vi "Safety_Check.vi"(0 "Duty No":u16 format="%.0b", 1 "Values":dbl[](array[numeric]) format="%.2f", 2 "Ch Names":string[](array[string]), 3 "Adam Loop Count":i32, 4 "Current Time":dbl) -> (5 "Scan comment":string)   [LabVIEW 2022 SP3]
uses:
  ADAM Client/Sub VIs/ADAM Controls/Update_scan_value.ctl
  Anemometry/Anemometry Sub Vis/Controls/In_Range.ctl
  ADAM Client/Sub VIs/Channel_State_Control.ctl
  Anemometry/Anemometry Sub Vis/Globals/Gas_management_global.vi
  ADAM_Global.vi
  Anemometry/Anemometry Sub Vis/Globals/EnFlo_Tunnel_Global.vi
panel:
  in  "Valve Tolerance":dbl=0.07
  in  "Minimum St Dev for Ozone inst":dbl=0.3
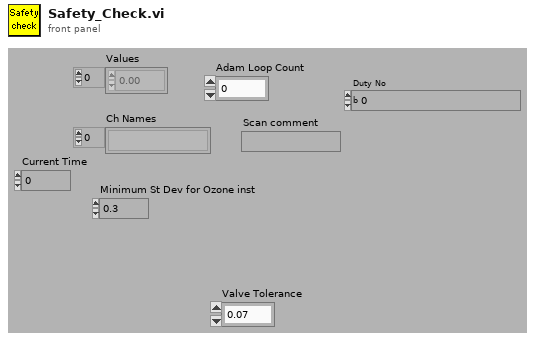
[diagram p1: front panel]
types:
  T1 = typedef "Update_scan_value.ctl" = cluster{"Channel Name":string, "New Value":dbl, "!Auto_Off":bool}
  T2 = enum16{"Append to Global", "Read Global then Clear"}
  T3 = enum16{"On", "Off", "Always On", "Always Off", "Delete"}
  T4 = typedef "In_Range.ctl" = enum16{"%", "±", "% & ±"}
  T5 = typedef "Channel_State_Control.ctl" = enum16{"Channel Name", "Channel Name Starts with", "Main Address"}
  T6 = cluster{"Bus Bar":string, "Connected Items":string[]}
  T7 = cluster{"Bus Bar":string, "Connected Items":string[]}[]
  T8 = typedef "LVDateTimeRec.ctl" = cluster{"fractional second":dbl, "second":i32, "minute":i32, "hour":i32, "day of month":i32, "month":i32, "year":i32, "day of week":i32, "day of year":i32, "DST":i32}
  T9 = typedef "Ch_description_ADAM.ctl" = cluster{"Ch Name":string, "Type":T10, "Function":T11, "Ch State":T12, "Calibration type":T13, "A":dbl, "B":dbl, "C":dbl, "D":dbl, "Comments":string, "Address":T14, "String":string, "Duty":u16}
  T10 = typedef "Module_type_ADAM.ctl" = string
  T11 = typedef "Function_ADAM.ctl" = enum16{"Analogue Input", "Digital Input", "Event counter", "Event rate", "Analogue Output", "Digital Output", "Relay Output"}
  T12 = typedef "Channel_State.ctl" = enum16{"On", "Off", "Always On", "Always Off"}
  T13 = typedef "Calib_type_ADAM.ctl" = string
  T14 = typedef "Address.ctl" = cluster{"Main":i32, "Ch.":i32, "Sub":i32, "Port Name":string}
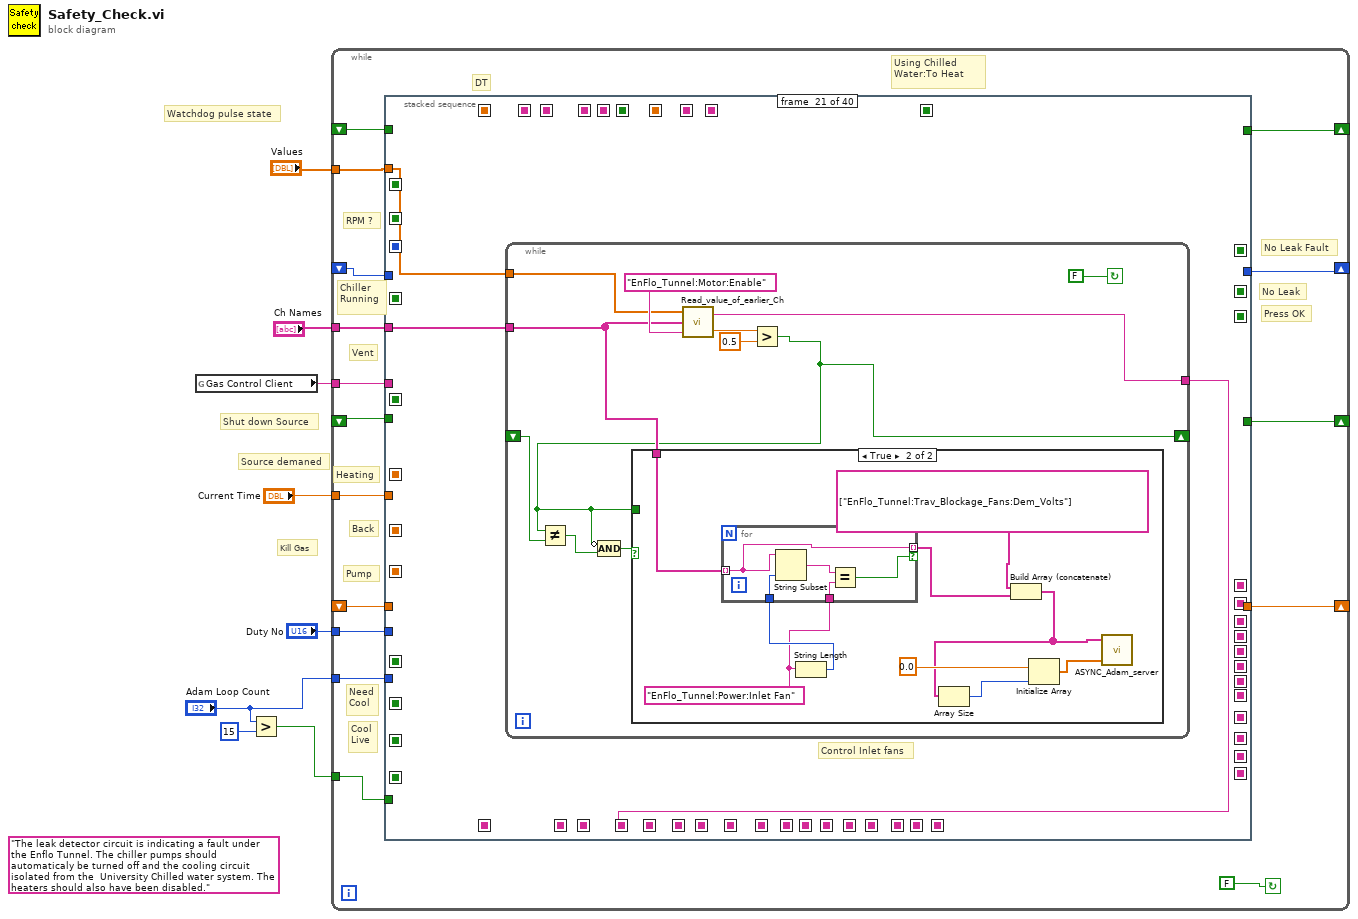
[diagram p0: block diagram]
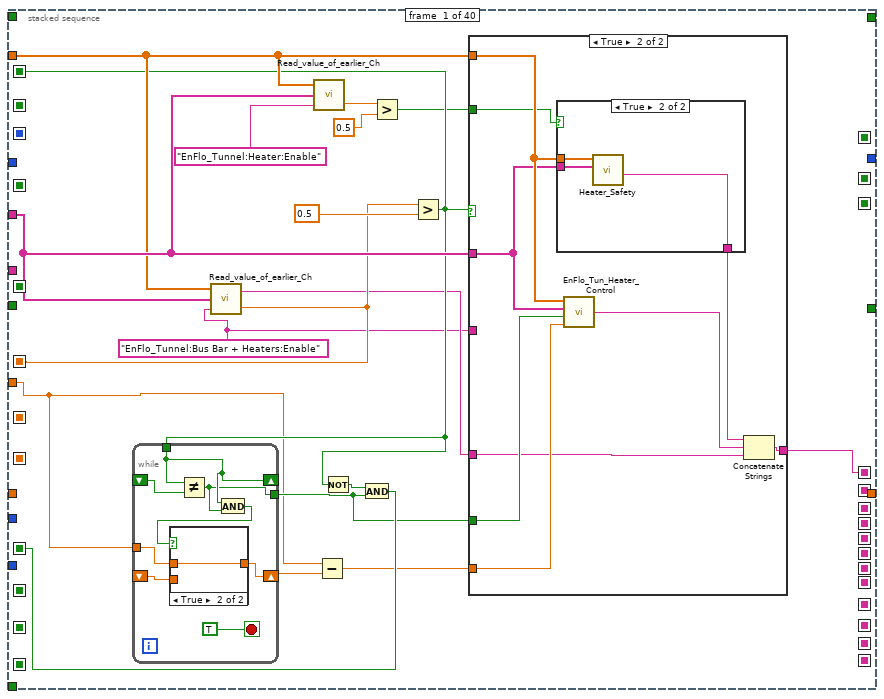
[diagram p2: hidden frame]
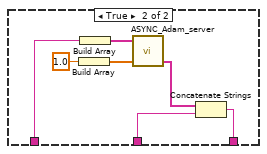
[diagram p5: hidden frame]
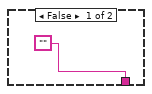
[diagram p6: hidden frame]
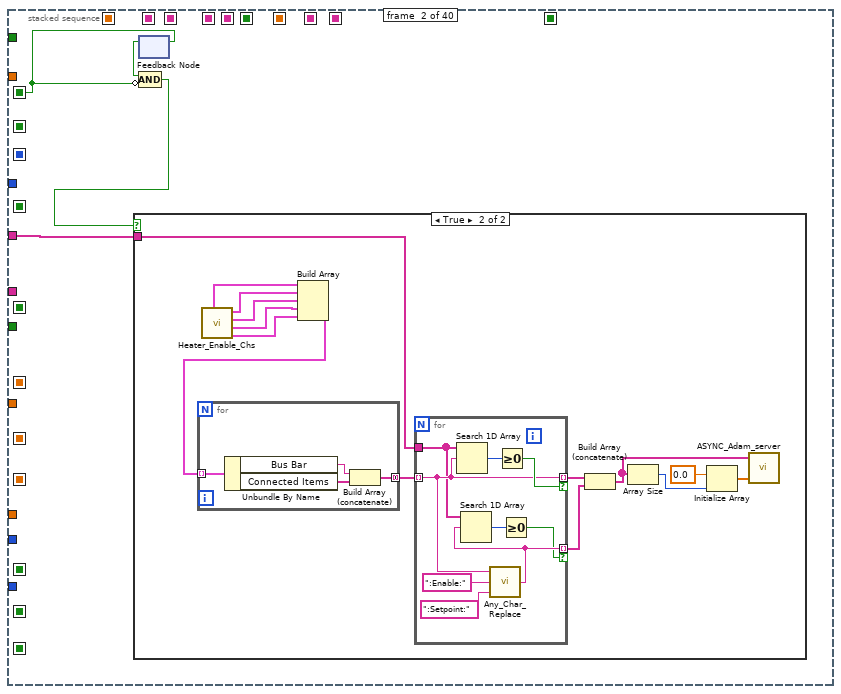
[diagram p7: hidden frame]
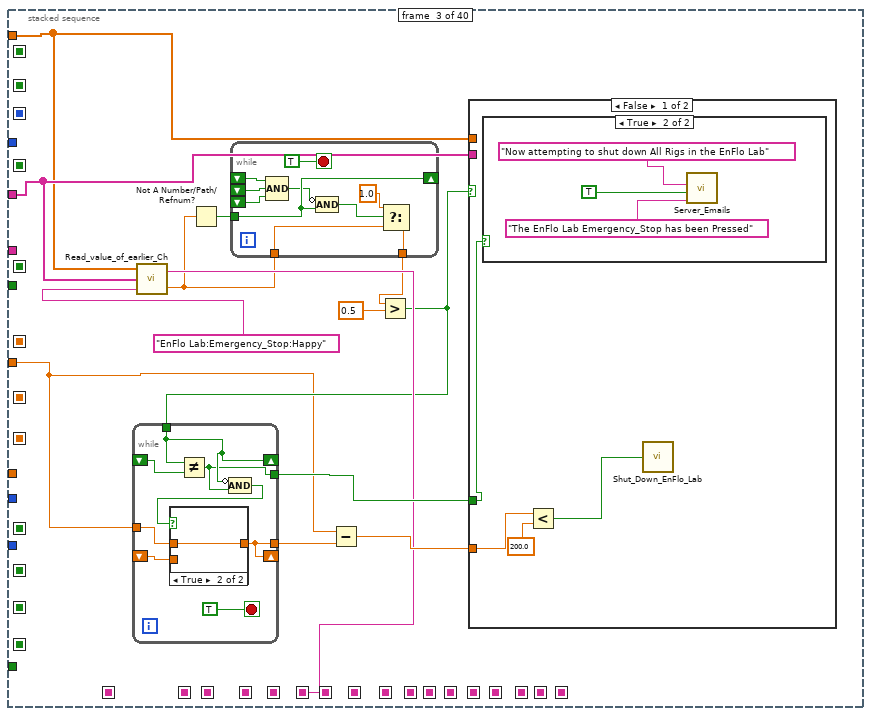
[diagram p9: hidden frame]
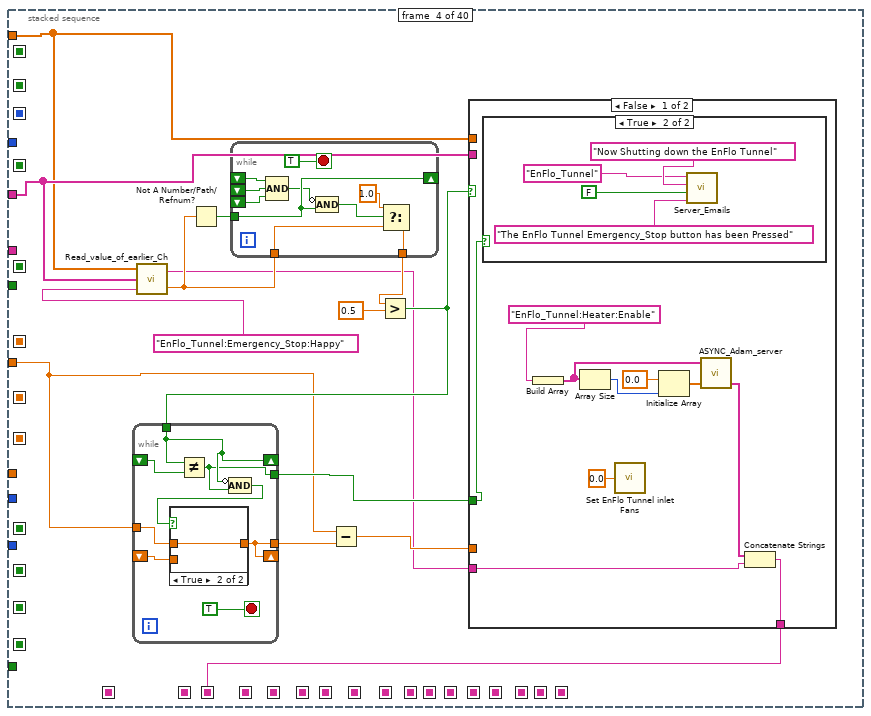
[diagram p13: hidden frame]
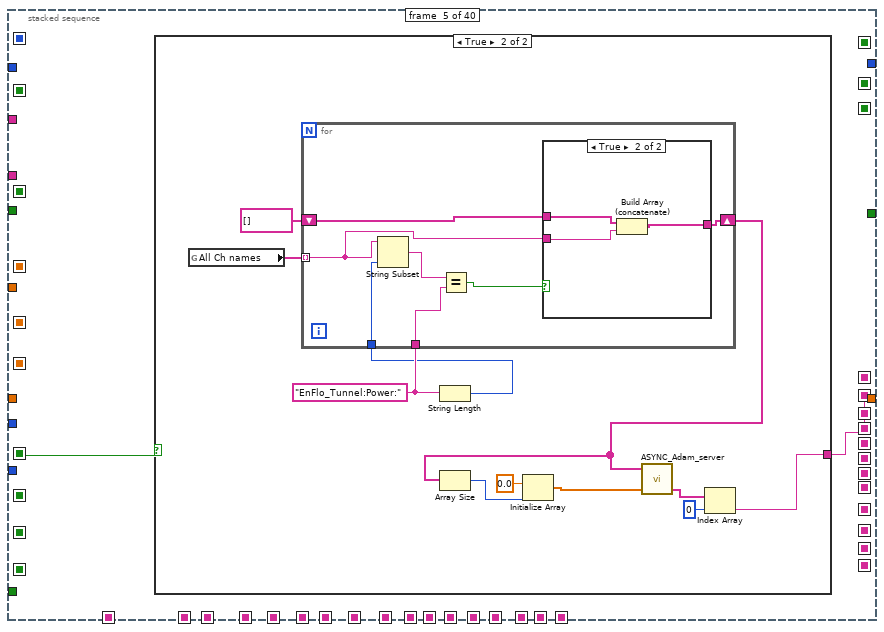
[diagram p17: hidden frame]
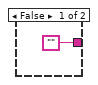
[diagram p18: hidden frame]
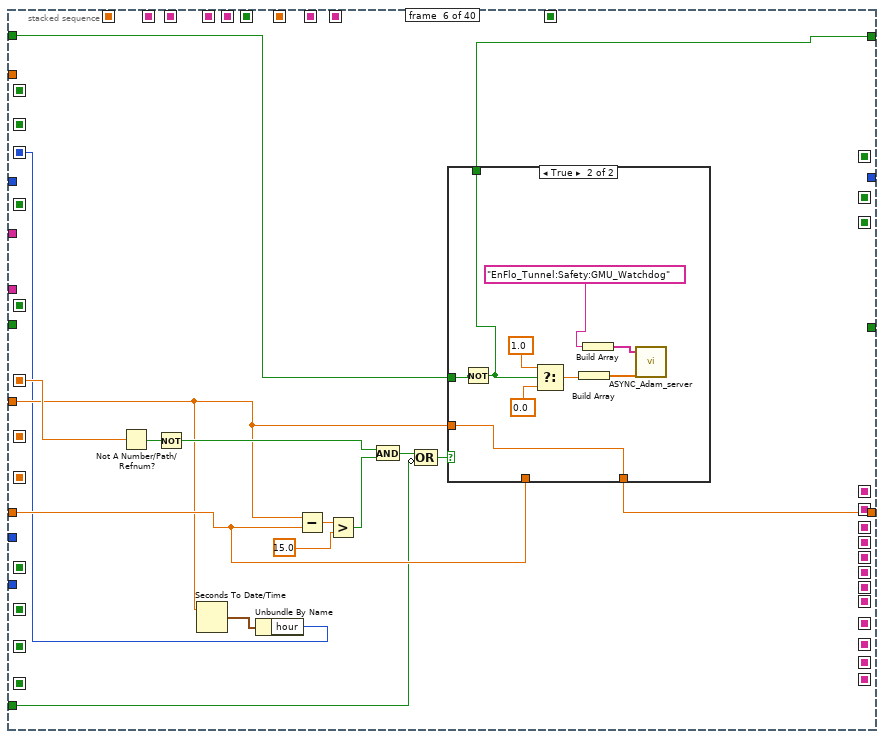
[diagram p20: hidden frame]
diagram:
  (unwired) "The leak detector circuit is indicating a fault under the Enflo Tunnel. The chiller pumps should automaticaly be turned off and the cooling circuit isolated from the  University Chilled water system. The heaters should also have been disabled." ("Message")
  # "Shut down Source"
  # "Source demaned"
  # "Watchdog pulse state"
  # "Kill Gas"
  n1 = global read "Gas_management_global.vi" "Gas Control Client"() -> (w6:string)
  n2 = Greater?(x="Adam Loop Count", y=15) -> (0:w4:bool)
  n3 = while {
    shift-left: _ -> [w19]
    shift-right: [w18] -> _
    shift-left: _ -> [w21]
    shift-right: [w20] -> _
    tunnel: w6 -> [w23]
    tunnel: "Ch Names" -> [w24]
    tunnel: "Values" -> [w22]
    shift-right: [w16] -> _
    shift-left: _ -> [w15]
    tunnel: w4 -> [w14]
    tunnel: "Current Time" -> [w13]
    tunnel: "Adam Loop Count" -> [w12]
    shift-right: [w11] -> _
    shift-left: _ -> [w10]
    tunnel: "Duty No" -> [w9]
    stop <- FALSE continue-if-true
    # "No Leak Fault"
    # "DT"
    # "Using Chilled Water:To Heat"
    # "Chiller Running"
    # "Back"
    # "Cool\nLive"
    # "RPM ?"
    # "Pump"
    # "Need\nCool"
    # "Heating"
    # "Vent"
    # "Press OK"
    # "No Leak"
    n4 = stacked-sequence {
      seq-local: [_ _ _ _ _ _ _ _ _ w383 _ _ _ _ _ _ _ _ _ _ _ _ _ _ _ _ _ _ _ _ _ _ _ _ _ _ _ _ _ _] -> [_ _ _ _ _ _ _ _ _ _ _ _ w464 w493 _ _ _ _ _ _ _ _ _ _ _ _ _ _ _ _ _ _ _ _ _ _ _ _ _ _]
      seq-local: [w38 _ _ _ _ _ _ _ _ _ _ _ _ _ _ _ _ _ _ _ _ _ _ _ _ _ _ _ _ _ _ _ _ _ _ _ _ _ _ _] -> [_ _ _ _ w199 _ _ _ _ _ _ _ _ _ _ _ _ _ _ _ _ _ _ _ _ _ _ _ _ _ _ _ _ _ _ _ _ _ _ _]
      seq-local: [_ _ _ _ _ _ _ _ _ _ _ _ _ _ _ _ _ _ _ _ _ _ _ _ _ _ _ _ _ w1044 _ _ _ _ _ _ _ _ _ _] -> [_ _ _ _ _ _ _ _ _ _ _ _ _ _ _ _ _ _ _ _ _ _ _ _ _ _ _ _ _ _ _ _ _ _ w1256 _ _ _ _ _]
      seq-local: [w30 _ _ _ _ _ _ _ _ _ _ _ _ _ _ _ _ _ _ _ _ _ _ _ _ _ _ _ _ _ _ _ _ _ _ _ _ _ _ _] -> [_ _ _ _ _ _ _ _ _ _ _ _ _ _ _ _ _ _ _ _ _ _ _ _ _ _ _ _ _ _ _ _ _ _ _ _ _ _ _ w1606]
      seq-local: [_ _ _ _ w198 _ _ _ _ _ _ _ _ _ _ _ _ _ _ _ _ _ _ _ _ _ _ _ _ _ _ _ _ _ _ _ _ _ _ _] -> [_ _ _ _ _ _ _ _ _ _ _ _ _ _ _ _ _ _ _ _ _ _ _ _ _ _ _ _ _ _ _ _ _ _ _ _ _ _ _ w1639]
      seq-local: [_ _ _ _ _ _ w250 _ _ _ _ _ _ _ _ _ _ _ _ _ _ _ _ _ _ _ _ _ _ _ _ _ _ _ _ _ _ _ _ _] -> [_ _ _ _ _ _ _ _ _ _ _ _ _ _ _ _ _ _ _ _ _ _ _ _ _ _ _ _ _ _ _ _ _ _ _ _ _ _ _ w1638]
      seq-local: [_ _ _ _ _ _ _ w333 _ _ _ _ _ _ _ _ _ _ _ _ _ _ _ _ _ _ _ _ _ _ _ _ _ _ _ _ _ _ _ _] -> [_ _ _ _ _ _ _ _ _ _ _ _ _ _ _ _ _ _ _ _ _ _ _ _ _ _ _ _ _ _ _ _ _ _ _ _ _ _ _ w1637]
      seq-local: [_ _ _ _ _ _ _ _ w355 _ _ _ _ _ _ _ _ _ _ _ _ _ _ _ _ _ _ _ _ _ _ _ _ _ _ _ _ _ _ _] -> [_ _ _ _ _ _ _ _ _ _ _ _ _ _ _ _ _ _ _ _ _ _ _ _ _ _ _ _ _ _ _ _ _ _ _ _ _ _ _ w1636]
      seq-local: [_ _ _ _ _ _ _ _ _ w384 _ _ _ _ _ _ _ _ _ _ _ _ _ _ _ _ _ _ _ _ _ _ _ _ _ _ _ _ _ _] -> [_ _ _ _ _ _ _ _ _ _ _ _ _ _ _ _ _ _ _ _ _ _ _ _ _ _ _ _ _ _ _ _ _ _ _ _ _ _ _ w1635]
      seq-local: [_ _ _ _ _ _ _ _ _ _ _ _ _ _ w526 _ _ _ _ _ _ _ _ _ _ _ _ _ _ _ _ _ _ _ _ _ _ _ _ _] -> [_ _ _ _ _ _ _ _ _ _ _ _ _ _ _ _ _ _ _ _ _ _ _ _ _ _ _ _ _ _ _ _ _ _ _ _ _ _ _ w1634]
      seq-local: [_ _ _ _ _ _ _ _ _ _ _ _ _ _ _ _ w614 _ _ _ _ _ _ _ _ _ _ _ _ _ _ _ _ _ _ _ _ _ _ _] -> [_ _ _ _ _ _ _ _ _ _ _ _ _ _ _ _ _ _ _ _ _ _ _ _ _ _ _ _ _ _ _ _ _ _ _ _ _ _ _ w1627]
      seq-local: [_ _ _ _ _ _ _ _ _ _ _ _ _ _ _ _ _ _ w693 _ _ _ _ _ _ _ _ _ _ _ _ _ _ _ _ _ _ _ _ _] -> [_ _ _ _ _ _ _ _ _ _ _ _ _ _ _ _ _ _ _ _ _ _ _ _ _ _ _ _ _ _ _ _ _ _ _ _ _ _ _ w1626]
      seq-local: [_ _ _ _ _ _ _ _ _ _ _ _ w466 _ _ _ _ _ _ _ _ _ _ _ _ _ _ _ _ _ _ _ _ _ _ _ _ _ _ _] -> [_ _ _ _ _ _ _ _ _ _ _ _ _ _ _ _ _ _ _ _ _ _ _ _ _ _ _ _ _ _ _ _ _ _ _ _ _ _ _ w1629]
      seq-local: [_ _ _ _ _ _ _ _ _ _ _ _ _ _ _ _ _ _ _ _ _ _ _ _ _ _ _ _ _ _ w1083 _ _ _ _ _ _ _ _ _] -> [_ _ _ _ _ _ _ _ _ _ _ _ _ _ _ _ _ _ _ _ _ _ _ _ _ _ _ _ _ _ _ _ _ _ _ _ _ _ _ w1630]
      seq-local: [_ _ _ _ _ _ _ _ _ _ _ _ _ _ _ _ _ _ _ _ _ _ _ _ _ _ w893 _ _ _ _ _ _ _ _ _ _ _ _ _] -> [_ _ _ _ _ _ _ _ _ _ _ _ _ _ _ _ _ _ _ _ _ _ _ _ _ _ _ _ _ _ _ _ _ _ _ _ _ _ _ w1615]
      seq-local: [_ _ _ _ _ _ _ _ _ _ _ _ _ _ _ _ _ _ _ _ _ _ _ w780 _ _ _ _ _ _ _ _ _ _ _ _ _ _ _ _] -> [_ _ _ _ _ _ _ _ _ _ _ _ _ _ _ _ _ _ _ _ _ _ _ _ _ _ _ _ _ _ _ _ _ _ _ _ _ _ _ w1631]
      seq-local: [_ _ _ _ _ _ _ _ _ _ _ _ _ _ _ _ _ _ _ _ _ _ _ _ _ _ _ _ _ _ _ _ _ w1217 _ _ _ _ _ _] -> [_ _ _ _ _ _ _ _ _ _ _ _ _ _ _ _ _ _ _ _ _ _ _ _ _ _ _ _ _ _ _ _ _ _ _ _ _ _ _ w1632]
      seq-local: [_ _ _ _ _ _ _ _ _ _ _ _ _ _ _ _ _ _ _ _ _ _ _ _ _ _ _ _ _ _ _ _ _ _ w1254 _ _ _ _ _] -> [_ _ _ _ _ _ _ _ _ _ _ _ _ _ _ _ _ _ _ _ _ _ _ _ _ _ _ _ _ _ _ _ _ _ _ _ _ _ _ w1633]
      seq-local: [w39 _ _ _ _ _ _ _ _ _ _ _ _ _ _ _ _ _ _ _ _ _ _ _ _ _ _ _ _ _ _ _ _ _ _ _ _ _ _ _] -> [_ _ _ _ _ w231 _ _ _ _ _ _ _ _ _ _ _ _ _ _ _ _ _ _ _ _ _ _ _ _ _ _ w1168 _ _ _ _ _ _ _]
      seq-local: [_ _ _ _ _ _ _ _ _ _ _ w428 _ _ _ _ _ _ _ _ _ _ _ _ _ _ _ _ _ _ _ _ _ _ _ _ _ _ _ _] -> [_ _ _ _ _ _ _ _ _ _ _ _ w463 _ _ _ _ _ _ _ _ _ _ _ _ _ _ _ _ _ _ _ _ _ _ _ _ _ _ _]
      seq-local: [_ _ _ _ _ _ _ _ _ _ _ w427 _ _ _ _ _ _ _ _ _ _ _ _ _ _ _ _ _ _ _ _ _ _ _ _ _ _ _ _] -> [_ _ _ _ _ _ _ _ _ _ _ _ _ _ _ _ _ _ _ _ _ _ _ _ _ _ _ _ _ _ _ _ _ _ _ _ _ _ _ w1625]
      seq-local: [_ _ _ _ _ _ _ _ _ _ _ _ _ _ _ _ _ _ _ _ _ _ _ _ _ _ _ w967 _ _ _ _ _ _ _ _ _ _ _ _] -> [_ _ _ _ _ _ _ _ _ _ _ _ _ _ _ _ _ _ _ _ _ _ _ _ _ _ _ _ _ _ _ _ _ _ _ _ _ _ _ w1623]
      seq-local: [_ _ _ _ _ _ _ _ _ _ _ _ _ _ _ _ _ w645 _ _ _ _ _ _ _ _ _ _ _ _ _ _ _ _ _ _ _ _ _ _] -> [_ _ _ _ _ _ _ _ _ _ _ _ _ _ _ _ _ _ _ _ _ _ _ _ _ _ _ _ _ _ _ _ _ _ _ _ _ _ _ w1624]
      seq-local: [_ _ _ _ _ _ _ _ _ _ _ _ _ _ _ _ _ _ _ _ _ _ _ _ w815 _ _ _ _ _ _ _ _ _ _ _ _ _ _ _] -> [_ _ _ _ _ _ _ _ _ _ _ _ _ _ _ _ _ _ _ _ _ _ _ _ _ _ _ _ _ _ _ _ _ _ _ _ _ _ _ w1613]
      seq-local: [_ _ w116 _ _ _ _ _ _ _ _ _ _ _ _ _ _ _ _ _ _ _ _ _ _ _ _ _ _ _ _ _ _ _ _ _ _ _ _ _] -> [_ _ _ _ _ _ _ _ _ _ _ _ _ _ _ _ _ _ _ _ _ _ _ _ _ _ _ _ _ _ _ _ _ _ _ _ _ _ _ w1622]
      seq-local: [_ _ _ _ _ _ _ _ _ _ _ _ _ _ _ _ _ _ _ _ _ _ _ _ _ _ _ _ _ _ _ _ _ _ _ w1280 _ _ _ _] -> [_ _ _ _ _ _ _ _ _ _ _ _ _ _ _ _ _ _ _ _ _ _ _ _ _ _ _ _ _ _ _ _ _ _ _ _ _ _ _ w1621]
      seq-local: [_ _ _ _ _ _ _ _ _ _ _ _ _ _ _ _ _ _ _ _ w720 _ _ _ _ _ _ _ _ _ _ _ _ _ _ _ _ _ _ _] -> [_ _ _ _ _ _ _ _ _ _ _ _ _ _ _ _ _ _ _ _ _ _ _ _ _ _ _ _ _ _ _ _ _ _ _ _ _ _ _ w1620]
      seq-local: [w33 _ _ _ _ _ _ _ _ _ _ _ _ _ _ _ _ _ _ _ _ _ _ _ _ _ _ _ _ _ _ _ _ _ _ _ _ _ _ _] -> [_ w80 _ _ _ _ _ _ _ _ _ _ _ _ _ _ _ _ _ _ _ _ _ _ _ _ _ _ _ _ w1082 w1096 _ _ _ _ _ _ _ _]
      seq-local: [_ _ _ _ _ _ _ _ _ _ _ _ _ _ _ _ _ _ _ _ _ _ _ _ _ _ _ _ _ _ _ w1094 _ _ _ _ _ _ _ _] -> [_ _ _ _ _ _ _ _ _ _ _ _ _ _ _ _ _ _ _ _ _ _ _ _ _ _ _ _ _ _ _ _ _ _ _ _ _ _ _ w1619]
      seq-local: [_ _ _ _ _ _ _ _ _ _ _ _ _ _ _ _ _ _ _ _ _ _ _ w781 _ _ _ _ _ _ _ _ _ _ _ _ _ _ _ _] -> [_ _ _ _ _ _ _ _ _ _ _ _ _ _ _ _ _ _ _ _ _ _ _ _ w808 _ _ _ _ w1042 _ _ w1163 _ _ _ _ _ _ _]
      seq-local: [_ _ _ _ _ _ _ _ _ _ _ _ _ _ _ _ _ _ _ _ _ _ _ _ _ _ _ _ _ _ _ _ w1155 _ _ _ _ _ _ _] -> [_ _ _ _ _ _ _ _ _ _ _ _ _ _ _ _ _ _ _ _ _ _ _ _ _ _ _ _ _ _ _ _ _ _ _ _ _ _ _ w1618]
      seq-local: [_ _ _ _ _ _ _ _ _ _ _ _ _ _ _ _ _ _ _ _ _ _ _ _ w817 _ _ _ _ _ _ _ _ _ _ _ _ _ _ _] -> [_ _ _ _ _ _ _ _ _ _ _ _ _ _ _ _ _ _ _ _ _ _ _ _ _ _ w895 _ _ _ _ _ _ _ _ _ _ _ w1392 _]
      seq-local: [_ _ _ _ _ _ _ _ _ _ _ _ _ _ _ _ _ _ _ w715 _ _ _ _ _ _ _ _ _ _ _ _ _ _ _ _ _ _ _ _] -> [_ _ _ _ _ _ _ _ _ _ _ _ _ _ _ _ _ _ _ _ _ _ w759 _ w816 _ _ _ _ w1039 _ _ _ _ _ _ _ _ _ _]
      seq-local: [_ _ _ _ _ _ _ _ _ _ _ _ _ _ _ _ _ _ _ _ _ _ _ _ _ _ _ _ _ _ _ _ _ _ _ _ w1311 _ _ _] -> [_ _ _ _ _ _ _ _ _ _ _ _ _ _ _ _ _ _ _ _ _ _ _ _ _ _ _ _ _ _ _ _ _ _ _ _ _ _ _ w1617]
      seq-local: [_ _ _ _ _ _ _ _ _ _ _ _ _ _ _ _ _ _ _ _ _ _ _ _ _ _ _ w966 _ _ _ _ _ _ _ _ _ _ _ _] -> [_ _ _ _ _ _ _ _ _ _ _ _ _ _ _ _ _ _ _ _ _ _ _ _ _ _ _ _ _ _ _ _ w1127 _ _ _ _ _ _ _]
      seq-local: [_ _ _ _ _ _ _ _ _ _ _ _ _ _ _ _ _ _ _ _ _ _ _ _ _ _ _ w965 _ _ _ _ _ _ _ _ _ _ _ _] -> [_ _ _ _ _ _ _ _ _ _ _ _ _ _ _ _ _ _ _ _ _ _ _ _ _ _ _ _ _ _ _ _ w1162 _ _ _ _ _ _ _]
      seq-local: [_ _ _ _ _ _ _ _ _ _ _ _ _ w494 _ _ _ _ _ _ _ _ _ _ _ _ _ _ _ _ _ _ _ _ _ _ _ _ _ _] -> [_ _ _ _ _ _ _ _ _ _ _ _ _ _ _ _ _ _ _ _ _ _ _ _ _ _ _ _ _ _ _ _ _ _ _ _ _ _ _ w1616]
      seq-local: [_ _ _ _ _ _ _ _ _ _ _ _ _ _ _ _ _ _ _ _ _ _ _ _ _ _ w894 _ _ _ _ _ _ _ _ _ _ _ _ _] -> [_ _ _ _ _ _ _ _ _ _ _ _ _ _ _ _ _ _ _ _ _ _ _ _ _ _ _ w964 w1028 w1040 _ _ w1160 _ _ _ _ _ _ _]
      seq-local: [_ _ _ _ _ _ _ _ _ _ _ _ _ _ _ _ _ _ _ _ _ _ _ _ _ _ _ _ _ w1041 _ _ _ _ _ _ _ _ _ _] -> [_ _ _ _ _ _ _ _ _ _ _ _ _ _ _ _ _ _ _ _ _ _ _ _ _ _ _ _ _ _ _ _ _ _ _ _ _ _ _ w1614]
      seq-local: [_ _ _ _ _ _ _ _ _ _ _ w426 _ _ _ _ _ _ _ _ _ _ _ _ _ _ _ _ _ _ _ _ _ _ _ _ _ _ _ _] -> [_ _ _ _ _ _ _ _ _ _ _ _ _ _ _ _ _ _ _ _ _ _ _ _ _ _ w892 _ _ _ _ _ _ _ _ _ _ _ _ _]
      seq-local: [_ _ _ _ _ _ _ _ _ _ _ _ _ _ _ w560 _ _ _ _ _ _ _ _ _ _ _ _ _ _ _ _ _ _ _ _ _ _ _ _] -> [_ _ _ _ _ _ _ _ _ _ _ _ _ _ _ _ _ _ _ _ _ _ _ _ _ _ _ _ _ _ _ _ _ _ _ _ _ _ _ w1612]
      seq-local: [_ _ _ _ _ _ _ _ _ _ _ _ _ _ _ _ _ _ _ _ _ _ _ _ w814 _ _ _ _ _ _ _ _ _ _ _ _ _ _ _] -> [_ _ _ _ _ _ _ _ _ _ _ _ _ _ _ _ _ _ _ _ _ _ _ _ _ w873 _ w963 w1029 _ _ _ w1126 _ _ _ _ _ w1390 _]
      seq-local: [_ _ _ _ _ _ _ _ _ _ _ _ _ _ _ _ _ _ _ _ _ _ _ _ _ _ _ _ w1017 _ _ _ _ _ _ _ _ _ _ _] -> [_ _ _ _ _ _ _ _ _ _ _ _ _ _ _ _ _ _ _ _ _ _ _ _ _ _ _ _ _ _ _ _ _ _ _ _ _ _ _ w1611]
      seq-local: [_ _ _ _ _ w226 _ _ _ _ _ _ _ _ _ _ _ _ _ _ _ _ _ _ _ _ _ _ _ _ _ _ _ _ _ _ _ _ _ _] -> [_ _ _ _ _ _ _ _ _ _ _ _ _ _ _ w559 _ _ _ _ _ _ _ _ _ _ _ _ _ _ _ _ _ _ _ _ _ _ _ _]
      seq-local: [_ _ _ _ _ _ _ _ _ _ _ w425 _ _ _ _ _ _ _ _ _ _ _ _ _ _ _ _ _ _ _ _ _ _ _ _ _ _ _ _] -> [_ _ _ _ _ _ _ _ _ _ _ _ _ _ _ _ _ _ _ _ _ _ _ _ w813 _ _ _ _ _ _ _ w1128 _ _ _ _ _ _ _]
      seq-local: [_ _ _ _ _ _ _ _ _ _ _ _ _ _ _ _ _ _ _ _ _ _ _ _ _ _ _ _ _ _ _ _ _ _ _ _ _ _ w1391 _] -> [_ _ _ _ _ _ _ _ _ _ _ _ _ _ _ _ _ _ _ _ _ _ _ _ _ _ _ _ _ _ _ _ _ _ _ _ _ _ _ w1610]
      seq-local: [_ _ _ _ _ _ _ _ _ _ _ _ _ _ _ _ _ _ _ _ _ w749 _ _ _ _ _ _ _ _ _ _ _ _ _ _ _ _ _ _] -> [_ _ _ _ _ _ _ _ _ _ _ _ _ _ _ _ _ _ _ _ _ _ w758 w779 w806 w872 _ _ _ _ _ _ _ _ _ _ _ _ _ _]
      seq-local: [_ _ _ _ _ _ _ _ _ _ _ _ _ _ _ _ _ _ _ _ _ w748 _ _ _ _ _ _ _ _ _ _ _ _ _ _ _ _ _ _] -> [_ _ _ _ _ _ _ _ _ _ _ _ _ _ _ _ _ _ _ _ _ _ _ _ _ _ _ _ _ _ _ _ _ _ _ _ _ _ _ w1609]
      seq-local: [_ _ _ _ _ _ _ _ _ _ _ _ _ _ _ _ _ _ _ _ _ _ _ _ _ w871 _ _ _ _ _ _ _ _ _ _ _ _ _ _] -> [_ _ _ _ _ _ _ _ _ _ _ _ _ _ _ _ _ _ _ _ _ _ _ _ _ _ _ _ _ _ _ _ _ _ _ _ _ _ _ w1608]
      seq-local: [_ _ _ _ _ _ _ _ _ _ _ _ _ _ _ _ _ _ _ _ _ _ w755 _ _ _ _ _ _ _ _ _ _ _ _ _ _ _ _ _] -> [_ _ _ _ _ _ _ _ _ _ _ _ _ _ _ _ _ _ _ _ _ _ _ w778 _ _ _ _ _ _ _ _ _ _ _ _ _ _ _ _]
      seq-local: [_ _ _ w149 _ _ _ _ _ _ _ _ _ _ _ _ _ _ _ _ _ _ _ _ _ _ _ _ _ _ _ _ _ _ _ _ _ _ _ _] -> [_ _ _ _ _ _ _ _ _ _ _ _ _ _ _ _ _ _ _ _ _ _ _ _ _ _ _ _ _ _ _ _ _ _ _ _ _ _ _ w1607]
      seq-local: [_ _ _ _ _ _ _ _ _ _ _ _ _ _ _ _ _ _ _ _ _ _ _ _ _ _ _ _ _ _ _ _ _ _ _ _ _ w1358 _ _] -> [_ _ _ _ _ _ _ _ _ _ _ _ _ _ _ _ _ _ _ _ _ _ _ _ _ _ _ _ _ _ _ _ _ _ _ _ _ _ _ w1605]
      seq-local: [_ _ _ _ _ _ _ _ _ _ w404 _ _ _ _ _ _ _ _ _ _ _ _ _ _ _ _ _ _ _ _ _ _ _ _ _ _ _ _ _] -> [_ _ _ _ _ _ _ _ _ _ _ _ _ _ _ _ _ _ _ _ _ _ _ _ _ _ _ _ _ _ _ _ _ _ _ _ _ _ _ w1604]
      seq-local: [_ _ _ _ _ _ _ _ _ _ w405 _ _ _ _ _ _ _ _ _ _ _ _ _ _ _ _ _ _ _ _ _ _ _ _ _ _ _ _ _] -> [_ _ _ _ _ _ _ _ _ _ _ _ w462 _ _ _ _ _ _ _ _ _ _ _ _ _ _ _ _ _ _ _ _ _ _ _ _ _ _ _]
      tunnel: w24 -> [w41 w78 w120 w161 _ _ w252 w340 w358 w385 w406 w429 w467 w495 w527 w561 w634 w646 w695 w717 w721 w750 w756 w782 w818 _ w896 w968 w1026 _ w1077 w1100 w1149 w1220 _ _ w1314 w1369 w1394 _]
      tunnel: w23 -> [_ _ _ _ _ _ w257 _ w369 _ _ _ _ _ _ _ _ _ _ _ _ _ _ _ _ _ _ _ _ _ _ _ _ _ _ _ _ _ _ _]
      tunnel: w22 -> [w40 _ w119 w160 _ _ w253 w336 w359 w386 w407 w430 w468 w496 w528 w562 w635 w647 w696 w718 w722 w751 w757 w783 w819 _ w897 w969 w1027 _ w1078 w1101 w1150 w1221 _ _ w1315 w1368 w1395 _]
      tunnel: w21 -> [_ _ _ _ _ w238 _ _ _ _ _ _ _ _ _ _ _ _ _ _ _ _ _ _ _ _ _ _ _ _ _ _ _ _ _ _ _ _ _ _]
      tunnel: [_ _ _ _ _ w237 _ _ _ _ _ _ _ _ _ _ _ _ _ _ _ _ _ _ _ _ _ _ _ _ _ _ _ _ _ _ _ _ _ _] -> w20
      tunnel: w19 -> [_ _ _ _ _ _ w256 _ _ _ _ _ _ _ _ _ _ _ _ _ _ _ _ _ _ _ _ _ _ _ _ _ _ _ _ _ _ _ _ _]
      tunnel: [_ _ _ _ _ _ w251 _ _ _ _ _ _ _ _ _ _ _ _ _ _ _ _ _ _ _ _ _ _ _ _ _ _ _ _ _ _ _ _ _] -> w18
      tunnel: [_ _ _ _ _ w236 _ _ _ _ _ _ _ _ _ _ _ _ _ _ _ _ _ _ _ _ _ _ _ _ _ _ _ _ _ _ _ _ _ _] -> w16
      tunnel: w15 -> [_ _ _ _ _ w233 _ _ _ _ _ _ _ _ _ _ _ _ _ _ _ _ _ _ _ _ _ _ _ _ _ _ _ _ _ _ _ _ _ _]
      tunnel: w14 -> [_ _ _ _ _ w224 _ _ _ _ _ _ _ _ _ w558 _ w643 w694 _ _ _ _ _ _ _ _ _ _ w1045 _ _ w1166 _ w1255 _ _ _ _ _]
      tunnel: w13 -> [w32 _ w109 w151 _ w227 _ _ _ _ _ _ _ _ _ _ _ w644 _ _ _ _ _ w777 _ _ _ _ _ _ _ _ _ _ _ _ w1313 _ w1393 _]
      tunnel: w12 -> [_ _ _ _ _ _ _ _ _ _ _ _ _ _ _ _ _ _ _ _ _ _ _ _ _ _ _ _ _ _ _ _ _ _ _ w1292 _ _ _ _]
      tunnel: [_ _ _ _ _ _ _ _ _ _ _ _ _ _ _ _ _ _ _ _ _ _ _ _ _ _ w891 _ _ _ _ _ _ _ _ _ _ _ _ _] -> w11
      tunnel: w10 -> [_ _ _ _ _ _ _ _ _ _ _ _ _ _ _ _ _ _ _ _ _ _ _ _ _ _ w890 _ _ _ _ _ _ _ _ _ _ _ _ _]
      tunnel: w9 -> [_ _ _ _ _ _ _ _ _ _ _ _ _ _ _ _ _ _ _ _ _ _ _ _ _ _ _ _ _ _ _ _ _ _ _ _ _ _ _ _]
      frame #0 {
        w25 = "EnFlo_Tunnel:Bus Bar + Heaters:Enable"
        n5 = call "Read_value_of_earlier_Ch.vi"("Desired Ch to Read"=w25, "Ch names"=w41, "Present scan array"=w40) -> ("Value"=w39:dbl, "Scan comment"=w31:string)  [unwired: 1 in]
        n6 = call "Read_value_of_earlier_Ch.vi"("Desired Ch to Read"="EnFlo_Tunnel:Heater:Enable", "Ch names"=w41, "Present scan array"=w40) -> ("Value"=w28:dbl)  [unwired: 1 in, 1 out]
        n7 = Greater?(x=w28, y=0.5) -> (0:w27:bool)
        n8 = Greater?(x=w39, y=0.5) -> (0:w33:bool)
        n9 = while {
          shift-right: [w48] -> _
          shift-left: _ -> [w50]
          tunnel: w33 -> [w48]
          tunnel: [w47] -> w36
          shift-right: [w45] -> w35
          shift-left: _ -> [w43]
          tunnel: w32 -> [w44]
          stop <- TRUE stop-if-true
          n10 = Not Equal?(x=w48, y=w50) -> (x != y?=w47:bool)
          n11 = And(x=w48, y=w47) -> (x .and. y?=w46:bool)
          n12 = case shown="True" w46 {
            tunnel: [w51 w52] -> w45
            tunnel: w44 -> [_ w52]
            tunnel: w43 -> [w51 _]
            frame False {
            }
            frame True {
            }
          }
        }
        n13 = Subtract(x=w32, y=w35) -> (x-y=w34:dbl)
        n14 = Not(x=w33) -> (.not. x?=w37:bool)
        n15 = And(x=w37, y=w36) -> (x .and. y?=w38:bool)
        n16 = case shown="True" w33 {
          tunnel: w40 -> [_ w71]
          tunnel: w41 -> [_ w70]
          tunnel: w36 -> [_ w73]
          tunnel: w34 -> [_ w72]
          tunnel: w31 -> [w54 w68]
          tunnel: [w53 w67] -> w30
          tunnel: w27 -> [w56 w66]
          tunnel: w25 -> [w55 _]
          frame False {
            n17 = case shown="False" w56 {
              tunnel: w55 -> [_ w63]
              tunnel: w54 -> [w57 w59]
              tunnel: [w57 w58] -> w53
              frame False {
              }
              frame True {
                n18 = Build Array(1.0 ("element")) -> (w62:dbl[])
                n19 = Build Array(w63) -> (w64:string[])
                n20 = call "ASYNC_Adam_server.vi"("Values"=w62, "Channel Names"=w64) -> ("Scan Comments"=w60:string[])  [unwired: 1 in, 2 out]
                n21 = Concatenate Strings(w60, w59) -> (w58:string)
              }
            }
          }
          frame True {
            n22 = case shown="True" w66 {
              tunnel: w71 -> [_ w77]
              tunnel: w70 -> [_ w76]
              tunnel: ["" w75] -> w65
              frame False {
              }
              frame True {
                n23 = call "Heater_Safety.vi"("Ch Names"=w76, "Values"=w77) -> ("Error String"=w75:string)  [unwired: 1 in, 4 out]
              }
            }
            n24 = call "EnFlo_Tun_Heater_Control.vi"("Heaters Enabled time (s)"=w72, "Heaters Just Enabled"=w73, "Ch Names"=w70, "Values"=w71) -> ("Error String"=w69:string)
            n25 = Concatenate Strings(w65, w69, w68) -> (w67:string)
          }
        }
      }
      frame #1 {
        n26 = feedback-in #1(w80) -> ()
        n27 = feedback #1() -> (w81:bool)  [unwired: 1 in]
        n28 = Compound Arithmetic op=AND(w81, invert w80) -> (w79:bool)
        n29 = case shown="True" w79 {
          tunnel: w78 -> [_ w84]
          frame False {
          }
          frame True {
            n30 = call "Heater_Enable_Chs.vi"() -> ("Bus Bar 4"=w95:T6, "Bus Bar 3"=w94:T6, "Bus Bar 2"=w93:T6, "Bus Bar 1"=w92:T6, "Inlet Heaters"=w91:T6)  [unwired: 4 in, 1 out]
            n31 = Build Array(w91, w92, w93, w94, w95) -> (w85:T7)
            n32 = for {
              tunnel: w85 -> [w108] mode=indexing
              tunnel: [w105] -> w83 mode=concatenating
              n33 = Unbundle By Name(w108) -> ("Bus Bar"=w107:string, "Connected Items"=w106:string[])
              n34 = Build Array (concatenate)(w107, w106) -> (w105:string[])
            }
            n35 = for {
              tunnel: w83 -> [w102] mode=indexing
              tunnel: w84 -> [w98]
              tunnel: [w102] -> w90 mode=indexing if=w103
              tunnel: [w97] -> w82 mode=indexing if=w96
              n36 = Search 1D Array(1D array=w98, element=w102) -> (index of element=w104:i32)  [unwired: 1 in]
              n37 = call "Any_Char_Replace.vi"("Replace with"=":Setpoint:", "Characters to replace"=":Enable:", "String in"=w102) -> ("String out"=w97:string)
              n38 = Search 1D Array(1D array=w98, element=w97) -> (index of element=w99:i32)  [unwired: 1 in]
              n39 = Greater Or Equal To 0?(x=w104) -> (x >= 0?=w103:bool)
              n40 = Greater Or Equal To 0?(x=w99) -> (x >= 0?=w96:bool)
            }
            n41 = Build Array (concatenate)(w90, w82) -> (w86:string[])
            n42 = Array Size(array=w86) -> (size(s)=w87:i32)
            n43 = Initialize Array(0.0, w87) -> (w89:dbl[])
            n44 = call "ASYNC_Adam_server.vi"("Values"=w89, "Channel Names"=w86) -> ()  [unwired: 1 in, 3 out]
          }
        }
      }
      frame #2 {
        n45 = call "Read_value_of_earlier_Ch.vi"("Desired Ch to Read"="EnFlo Lab:Emergency_Stop:Happy", "Ch names"=w120, "Present scan array"=w119) -> ("Value"=w114:dbl, "Scan comment"=w116:string)  [unwired: 1 in]
        n46 = Not A Number/Path/Refnum?(number/path/refnum=w114) -> (NaN/Path/Refnum?=w113:bool)
        n47 = while {
          tunnel: w114 -> [w124]
          shift-right: [w128] -> _
          shift-left: _ -> [w131]
          tunnel: w113 -> [w128]
          shift-left: _ -> [w130]
          shift-left: _ -> [w129]
          tunnel: [w123] -> w110
          stop <- TRUE stop-if-true
          n48 = Compound Arithmetic op=AND(w131, w130, w129) -> (w127:bool)
          n49 = Compound Arithmetic op=AND(invert w127, w128) -> (w126:bool)
          n50 = Select(t=1.0, s=w126, f=w124) -> (s? t:f=w123:dbl)
        }
        n51 = Greater?(x=w110, y=0.5) -> (0:w111:bool)
        n52 = while {
          shift-right: [w137] -> _
          shift-left: _ -> [w139]
          tunnel: w111 -> [w137]
          tunnel: [w136] -> w118
          shift-right: [w132] -> _
          shift-left: _ -> [w133]
          tunnel: w109 -> [w134]
          tunnel: [w132] -> w115
          stop <- TRUE stop-if-true
          n53 = Not Equal?(x=w137, y=w139) -> (x != y?=w136:bool)
          n54 = Compound Arithmetic op=AND(invert w137, w136) -> (w135:bool)
          n55 = case shown="True" w135 {
            tunnel: [w140 w141] -> w132
            tunnel: w134 -> [_ w141]
            tunnel: w133 -> [w140 _]
            frame False {
            }
            frame True {
            }
          }
        }
        n56 = Subtract(x=w109, y=w115) -> (x-y=w117:dbl)
        n57 = case shown="False" w111 {
          tunnel: w119 -> [_ _]
          tunnel: w120 -> [_ _]
          tunnel: w118 -> [w143 _]
          tunnel: w117 -> [w145 _]
          frame False {
            n58 = case shown="True" w143 {
              frame False {
              }
              frame True {
                n59 = call "Server_Emails.vi"("Message"="Now attempting to shut down All Rigs in the EnFlo Lab", "Contact All clients?"=TRUE, "Subject"="The EnFlo Lab Emergency_Stop has been Pressed") -> ()  [unwired: 2 in, 3 out]
              }
            }
            n60 = Less?(x=w145, y=200.0) -> (x < y?=w142:bool)
            n61 = call "Shut_Down_EnFlo_Lab.vi"("Initial Shutdown"=w142) -> ()
          }
          frame True {
          }
        }
      }
      frame #3 {
        n62 = call "Read_value_of_earlier_Ch.vi"("Desired Ch to Read"="EnFlo_Tunnel:Emergency_Stop:Happy", "Ch names"=w161, "Present scan array"=w160) -> ("Value"=w156:dbl, "Scan comment"=w150:string)  [unwired: 1 in]
        n63 = Not A Number/Path/Refnum?(number/path/refnum=w156) -> (NaN/Path/Refnum?=w155:bool)
        n64 = while {
          tunnel: w156 -> [w165]
          shift-right: [w169] -> _
          shift-left: _ -> [w172]
          tunnel: w155 -> [w169]
          shift-left: _ -> [w171]
          shift-left: _ -> [w170]
          tunnel: [w164] -> w152
          stop <- TRUE stop-if-true
          n65 = Compound Arithmetic op=AND(w172, w171, w170) -> (w168:bool)
          n66 = Compound Arithmetic op=AND(invert w168, w169) -> (w167:bool)
          n67 = Select(t=1.0, s=w167, f=w165) -> (s? t:f=w164:dbl)
        }
        n68 = Greater?(x=w152, y=0.5) -> (0:w153:bool)
        n69 = while {
          shift-right: [w178] -> _
          shift-left: _ -> [w180]
          tunnel: w153 -> [w178]
          tunnel: [w177] -> w159
          shift-right: [w173] -> _
          shift-left: _ -> [w174]
          tunnel: w151 -> [w175]
          tunnel: [w173] -> w157
          stop <- TRUE stop-if-true
          n70 = Not Equal?(x=w178, y=w180) -> (x != y?=w177:bool)
          n71 = Compound Arithmetic op=AND(invert w178, w177) -> (w176:bool)
          n72 = case shown="True" w176 {
            tunnel: [w181 w182] -> w173
            tunnel: w175 -> [_ w182]
            tunnel: w174 -> [w181 _]
            frame False {
            }
            frame True {
            }
          }
        }
        n73 = Subtract(x=w151, y=w157) -> (x-y=w158:dbl)
        n74 = case shown="False" w153 {
          tunnel: w160 -> [_ _]
          tunnel: w161 -> [_ _]
          tunnel: w159 -> [w192 _]
          tunnel: w158 -> [_ _]
          tunnel: w150 -> [w185 w197]
          tunnel: [w184 w197] -> w149
          frame False {
            n75 = case shown="True" w192 {
              frame False {
              }
              frame True {
                n76 = call "Server_Emails.vi"("Client Name Contains"="EnFlo_Tunnel", "Message"="Now Shutting down the EnFlo Tunnel", "Contact All clients?"=FALSE, "Subject"="The EnFlo Tunnel Emergency_Stop button has been Pressed") -> ()  [unwired: 1 in, 3 out]
              }
            }
            n77 = Build Array("EnFlo_Tunnel:Heater:Enable") -> (w188:string[])
            n78 = Array Size(array=w188) -> (size(s)=w189:i32)
            n79 = call "Set EnFlo Tunnel inlet Fans.vi"("Tunnel Velocity m/s"=0.0) -> ()  [unwired: 1 out]
            n80 = Initialize Array(0.0, w189) -> (w191:dbl[])
            n81 = call "ASYNC_Adam_server.vi"("Values"=w191, "Channel Names"=w188) -> ("Scan Comments"=w186:string[])  [unwired: 1 in, 2 out]
            n82 = Concatenate Strings(w186, w185) -> (w184:string)
          }
          frame True {
          }
        }
      }
      frame #4 {
        n83 = case shown="True" w199 {
          tunnel: ["" w202] -> w198
          frame False {
          }
          frame True {
            w211 = "EnFlo_Tunnel:Power:"
            n84 = global read "ADAM_Global.vi" "All Ch names"() -> (w201:string[])
            n85 = String Length(string=w211) -> (length=w210:i32)
            n86 = for {
              shift-right: [w213] -> w206
              shift-left: string[] [] -> [w214]
              tunnel: w201 -> [w217] mode=indexing
              tunnel: w210 -> [w218]
              tunnel: w211 -> [w215]
              n87 = String Subset(string=w217, length (rest)=w218) -> (substring=w216:string)  [unwired: 1 out]
              n88 = Equal?(x=w216, y=w215) -> (x = y?=w212:bool)
              n89 = case shown="True" w212 {
                tunnel: w217 -> [_ w222]
                tunnel: w214 -> [w219 w220]
                tunnel: [w219 w221] -> w213
                frame False {
                }
                frame True {
                  n90 = Build Array (concatenate)(w220, w222) -> (w221:string[])
                }
              }
            }
            n91 = Array Size(array=w206) -> (size(s)=w207:i32)
            n92 = Initialize Array(0.0 ("element"), w207) -> (w205:dbl[])
            n93 = call "ASYNC_Adam_server.vi"("Values"=w205, "Channel Names"=w206) -> ("Scan Comments"=w204:string[])  [unwired: 1 in, 2 out]
            n94 = Index Array(array=w204, index=0) -> (element=w202:string)
          }
        }
      }
      frame #5 {
        n95 = Not A Number/Path/Refnum?(number/path/refnum=w231) -> (NaN/Path/Refnum?=w230:bool)
        n96 = Not(x=w230) -> (.not. x?=w228:bool)
        n97 = Seconds To Date/Time(time stamp (now)=w227) -> (date time rec=w232:T8)  [unwired: 1 in]
        n98 = Unbundle By Name(w232) -> ("hour"=w226:i32)
        n99 = Subtract(x=w227, y=w233) -> (x-y=w235:dbl)
        n100 = Greater?(x=w235, y=15.0) -> (0:w229:bool)
        n101 = And(x=w228, y=w229) -> (x .and. y?=w225:bool)
        n102 = Compound Arithmetic op=OR(w225, invert w224) -> (w223:bool)
        n103 = case shown="True" w223 {
          tunnel: w238 -> [w239 w247]
          tunnel: [w239 w246] -> w237
          tunnel: [w240 w245] -> w236
          tunnel: w227 -> [_ w245]
          tunnel: w233 -> [w240 _]
          frame False {
          }
          frame True {
            n104 = Not(x=w247) -> (.not. x?=w246:bool)
            n105 = Select(t=1.0 ("Suction"), s=w246, f=0.0 ("Suction")) -> (s? t:f=w244:dbl)
            n106 = Build Array(w244) -> (w243:dbl[])
            n107 = Build Array("EnFlo_Tunnel:Safety:GMU_Watchdog" ("Desired Ch to Read")) -> (w242:string[])
            n108 = call "ASYNC_Adam_server.vi"("Values"=w243, "Channel Names"=w242) -> ()  [unwired: 2 in, 2 out]
          }
        }
      }
      frame #6 {
        n109 = call "Source_Q_wrong.vi"("Ch Names"=w252, "Values"=w253) -> ("Gas Error?"=w251:bool)  [unwired: 1 out]
        n110 = Compound Arithmetic op=AND(w251, invert w256) -> (w255:bool)
        n111 = case shown="True" w255 {
          tunnel: w257 -> [_ w263]
          tunnel: w253 -> [_ w262]
          tunnel: w252 -> [_ w261]
          tunnel: T1 {"Channel Name"="", "New Value"=0.0, "!Auto_Off"=FALSE} ("Update Scan Value Cluster") -> [_ w260]
          tunnel: ["" w259] -> w250
          frame False {
          }
          frame True {
            n112 = stacked-sequence {
              seq-local: [_ w295 _ _ _] -> [_ _ _ _ w328]
              seq-local: [w265 _ _ _ _] -> [_ _ _ _ w327]
              seq-local: [w264 _ _ _ _] -> [_ _ _ _ w326]
              seq-local: [_ w281 _ _ _] -> [_ _ _ _ w325]
              tunnel: w263 -> [_ _ w298 _ w329]
              tunnel: w262 -> [w275 w285 _ w307 _]
              tunnel: w261 -> [w276 w284 _ w308 _]
              tunnel: w260 -> [_ _ w297 w306 _]
              tunnel: [_ _ _ _ w324] -> w259
              frame #0 {
                n113 = Build Array("GMU:Carrier 1:Dem Volt", "GMU:Carrier 2:Dem Volt", "GMU:Trace:Dem Volt") -> (w277:string[])
                n114 = call "Read_Earlier_Channels.vi"("Present scan array"=w275, "Ch names"=w276, "Desired Channels"=w277) -> ("Scan comments"=w264:string, "Index 0"=w271:dbl, "Index 1"=w270:dbl, "Index 2"=w269:dbl)  [unwired: 2 out]
                n115 = Build Array(w271, w270, w269) -> (w268:dbl[])
                n116 = for {
                  tunnel: w268 -> [w280] mode=indexing
                  tunnel: 1e-05 -> [w279]
                  tunnel: [w278] -> w266 mode=indexing
                  n117 = Greater?(x=w280, y=w279) -> (0:w278:bool)
                }
                n118 = Or Array Elements(Boolean array=w266) -> (logical OR=w265:bool)
              }
              frame #1 {
                n119 = Build Array("GMU:Source:Dem Q", "GMU:Source:Dem Strength", "GMU:Source:Meas Q", "GMU:Source:Meas Strength") -> (w290:string[])
                n120 = call "Read_Earlier_Channels.vi"("Present scan array"=w285, "Ch names"=w284, "Desired Channels"=w290) -> ("Scan comments"=w281:string, "Index 0"=w289:dbl, "Index 1"=w288:dbl, "Index 2"=w287:dbl, "Index 3"=w286:dbl)  [unwired: 1 out]
                n121 = call "Read_value_of_earlier_Ch.vi"("Desired Ch to Read"="GMU:Detector:Strength", "Ch names"=w284, "Present scan array"=w285) -> ("Value"=w282:dbl)  [unwired: 1 in, 1 out]
                n122 = Format Into String(format string="Dem %.0f l/min %.2f%%, Meas %.0f l/min %.2f%% and the detector strength is %.2f%%. The source has been switched off" ("Format String"), w289, w288, w287, w286, w282) -> (resulting string=w295:string)  [unwired: 2 in, 1 out]
              }
              frame #2 {
                w299 = 0.0 ("Bundle Element")
                n123 = call "Shut_down_Hi_Tecs.vi"("Client Name"=w298) -> ()  [unwired: 6 out]
                n124 = Bundle By Name(cluster=w297, "Channel Name"="GMU:Source:Dem Q", "New Value"=w299) -> (w304:T1)
                n125 = Bundle By Name(cluster=w297, "Channel Name"="GMU:Source:Dem Strength", "New Value"=w299) -> (w305:T1)
                n126 = Build Array(w304, w305) -> (w301:T1[])
                n127 = call "Update_Current_Value_server.vi"("Mode"=T2."Append to Global", "Update array in"=w301) -> ()  [unwired: 1 in, 1 out]
              }
              frame #3 {
                n128 = for {
                  tunnel: w308 -> [w309] mode=indexing
                  tunnel: w307 -> [w315] mode=indexing
                  tunnel: w306 -> [w310]
                  n129 = Equal?(x=w315, y=2.0) -> (x = y?=w312:bool)
                  n130 = Match Pattern(string=w309, regular expression="Source:Status") -> (offset past match=w316:i32)  [unwired: 4 out]
                  n131 = Greater Or Equal To 0?(x=w316) -> (x >= 0?=w313:bool)
                  n132 = And(x=w312, y=w313) -> (x .and. y?=w311:bool)
                  n133 = case shown="True" w311 {
                    tunnel: w310 -> [w323 _]
                    tunnel: w309 -> [w322 _]
                    frame True {
                      n134 = Bundle By Name(cluster=w323, "Channel Name"=w322, "New Value"=0.0) -> (w320:T1)
                      n135 = Build Array(w320) -> (w319:T1[])
                      n136 = call "Update_Current_Value_server.vi"("Mode"=T2."Append to Global", "Update array in"=w319) -> ()  [unwired: 1 in, 1 out]
                    }
                    frame False {
                    }
                  }
                }
              }
              frame #4 {
                n137 = case shown="True" w327 {
                  tunnel: w329 -> [_ w332]
                  tunnel: w328 -> [_ w331]
                  frame False {
                  }
                  frame True {
                    n138 = call "Server_Emails.vi"("Client Name Contains"=w332, "Message"=w331, "Subject"="Source Off") -> ()  [unwired: 2 in, 3 out]
                  }
                }
                n139 = Concatenate Strings(w326, w325) -> (w324:string)
              }
            }
          }
        }
      }
      frame #7 {
        n140 = global read "ADAM_Global.vi" "Program Hung Clients"() -> (w341:string[])
        n141 = for {
          tunnel: w341 -> [w350] mode=indexing
          tunnel: w336 -> [w352]
          tunnel: w340 -> [w351]
          tunnel: [w348] -> w339 mode=indexing
          tunnel: [w345] -> w338 mode=indexing
          shift-right: [w343] -> w333
          shift-left: "" -> [w344]
          n142 = call "Split_Ch_name.vi"("Ch name"=w350) -> ("Low level"=w347:string)  [unwired: 2 out]
          n143 = call "Shut_Down_Client_Demands.vi"("Ch Names"=w351, "Values"=w352, "Client Name"=w350) -> ("Comments"=w342:string)
          n144 = Concatenate Strings(w344, w342) -> (w343:string)
          n145 = Concatenate Strings(w347, ":Source:Status") -> (w348:string)
          n146 = Concatenate Strings(w347, ":Program:Sync") -> (w345:string)
        }
        n147 = Build Array (concatenate)(w339, w338) -> (w337:string[])
        n148 = call "Cntrl_Ch_Status_low.vi"("Mode"=T3."Delete", "Channel names"=w337) -> ()  [unwired: 1 out]
      }
      frame #8 {
        n149 = call "Read_value_of_earlier_Ch.vi"("Desired Ch to Read"="GMU:Detector:Happy", "Ch names"=w358, "Present scan array"=w359) -> ("Value"=w362:dbl, "Scan comment"=w357:string)  [unwired: 1 in]
        n150 = feedback #2() -> (w364:dbl[])  [unwired: 1 in]
        n151 = Build Array (concatenate)(w362, w364) -> (w365:dbl[])
        n152 = global write "ADAM_Global.vi" "Program Hung Clients"(string[] [] ("Program Hung Clients")) -> ()
        n153 = Array Subset(array=w365, length=15) -> (w354:dbl[])  [unwired: 1 in]
        n154 = feedback-in #2(w354) -> ()
        n155 = call "Mean_fr_NaN_data.vi"("Data"=w354) -> ("Mean value"=w353:dbl)  [unwired: 1 out]
        n156 = Greater?(x=w353, y=0.5) -> (0:w361:bool)
        n157 = feedback #3() -> (w360:bool)  [unwired: 1 in]
        n158 = Compound Arithmetic op=AND(invert w361, w360) -> (w366:bool)
        n159 = case shown="True" w366 {
          tunnel: w369 -> [_ w379]
          tunnel: w359 -> [_ w378]
          tunnel: w358 -> [_ w377]
          tunnel: ["" w372] -> w356
          frame False {
          }
          frame True {
            n160 = call "Read_value_of_earlier_Ch.vi"("Desired Ch to Read"="EnFlo_Tunnel:Gas Solenoid:Status", "Ch names"=w377, "Present scan array"=w378) -> ("Value"=w374:dbl, "Scan comment"=w372:string)  [unwired: 1 in]
            n161 = Greater?(x=w374, y=0.5) -> (0:w373:bool)
            n162 = case shown="False" w373 {
              tunnel: w379 -> [w381 _]
              frame False {
                n163 = call "Server_Emails.vi"("Client Name Contains"=w381, "Message"="The GMU Gas detector IR2100 is unhappy. Please check concentrations etc. This will have turned off the gases from the outside bottle store.  You will need to repress the blue gas button after clearing the fault by purging the source with carrier gas only.", "Subject"="GMU Gas Detector Unhappy") -> ()  [unwired: 2 in, 3 out]
              }
              frame True {
              }
            }
          }
        }
        n164 = Concatenate Strings(w357, w356) -> (w355:string)
        n165 = feedback-in #3(w361) -> ()
      }
      frame #9 {
        n166 = while {
          tunnel: w386 -> [w400]
          tunnel: w385 -> [w399]
          shift-right: [w388] -> _
          shift-left: _ -> [w392]
          tunnel: [w393] -> w384
          shift-left: _ -> [w391]
          shift-left: _ -> [w390]
          shift-left: _ -> [w389]
          tunnel: [w387] -> w383
          stop <- FALSE continue-if-true
          n167 = call "Read_value_of_earlier_Ch.vi"("Desired Ch to Read"="EnFlo Lab:Leak_Detector:Happy", "Ch names"=w399, "Present scan array"=w400) -> ("Value"=w397:dbl, "Scan comment"=w393:string)  [unwired: 1 in]
          n168 = Greater?(x=w397, y=0.5) -> (0:w388:bool)
          n169 = Compound Arithmetic op=AND(invert w388, invert w392, invert w391, w390, w389) -> (w395:bool)
          n170 = case shown="True" w395 {
            frame False {
            }
            frame True {
              n171 = call "Server_Emails.vi"("Client Name Contains"="EnFlo_Tunnel", "Message"="The leak detector is indicating a leak under the Enflo Tunnel. The chiller pumps should automaticaly be turned off and the cooling circuit isolated from the  University Chilled water system. The heaters should also have been disabled.", "Subject"="Leak Detected under EnFlo Tunnel") -> ()  [unwired: 2 in, 3 out]
            }
          }
          n172 = Compound Arithmetic op=OR(w392, w391, w390, w389, w388) -> (w387:bool)
        }
      }
      frame #10 {
        n173 = while {
          tunnel: w407 -> [w421]
          tunnel: w406 -> [w420]
          shift-right: [w409] -> _
          shift-left: _ -> [w413]
          tunnel: [w414] -> w404
          shift-left: _ -> [w412]
          shift-left: _ -> [w411]
          shift-left: _ -> [w410]
          tunnel: [w408] -> w405
          stop <- FALSE continue-if-true
          n174 = call "Read_value_of_earlier_Ch.vi"("Desired Ch to Read"="EnFlo Lab:Leak_Detector_Circuit:Happy", "Ch names"=w420, "Present scan array"=w421) -> ("Value"=w418:dbl, "Scan comment"=w414:string)  [unwired: 1 in]
          n175 = Greater?(x=w418, y=0.5) -> (0:w409:bool)
          n176 = Compound Arithmetic op=AND(invert w409, invert w413, invert w412, w411, w410) -> (w416:bool)
          n177 = case shown="True" w416 {
            frame False {
            }
            frame True {
              n178 = call "Server_Emails.vi"("Client Name Contains"="EnFlo_Tunnel", "Message"="The leak detector circuit is indicating a fault under the Enflo Tunnel. The chiller pumps should automaticaly be turned off and the cooling circuit isolated from the  University Chilled water system. The heaters should also have been disabled.", "Subject"="Leak Detecter Circuit Fault under EnFlo Tunnel") -> ()  [unwired: 2 in, 3 out]
            }
          }
          n179 = Compound Arithmetic op=OR(w413, w412, w411, w410, w409) -> (w408:bool)
        }
      }
      frame #11 {
        n180 = while {
          tunnel: w430 -> [w435]
          tunnel: w429 -> [w434]
          shift-right: [w455] -> w428
          shift-left: _ -> [w456]
          tunnel: [w448] -> w427
          shift-right: [w440] -> _
          shift-left: _ -> [w439]
          tunnel: [w437] -> w426
          tunnel: [w436] -> w425
          stop <- FALSE continue-if-true
          n181 = call "Read_value_of_earlier_Ch.vi"("Desired Ch to Read"="EnFlo_Tunnel:Chiller_Pump:Enable", "Ch names"=w434, "Present scan array"=w435) -> ("Value"=w432:dbl, "Scan comment"=w431:string)  [unwired: 1 in]
          n182 = call "Read_value_of_earlier_Ch.vi"("Desired Ch to Read"="EnFlo_Tunnel:Chiller_Pump:Running", "Ch names"=w434, "Present scan array"=w435) -> ("Value"=w438:dbl, "Scan comment"=w449:string)  [unwired: 1 in]
          n183 = call "Read_value_of_earlier_Ch.vi"("Desired Ch to Read"="EnFlo_Tunnel:Chilled Water:Pressure_OK", "Ch names"=w434, "Present scan array"=w435) -> ("Value"=w447:dbl, "Scan comment"=w450:string)  [unwired: 1 in]
          n184 = feedback #4() -> (w444:dbl[])  [unwired: 1 in]
          n185 = call "Running_Ch_Average.vi"("Shift In"=w444, "History length"=10, "Reset Average after Seconds"=120.0, "New Value"=w447) -> ("Shift Out"=w445:dbl[], "mean"=w446:dbl)  [unwired: 1 in, 1 out]
          n186 = feedback-in #4(w445) -> ()
          n187 = Greater?(x=w446, y=0.5) -> (0:w455:bool)
          n188 = Greater?(x=w438, y=0.5) -> (0:w436:bool)
          n189 = Compound Arithmetic op=AND(invert w455, w456, w436) -> (w454:bool)
          n190 = case shown="True" w454 {
            frame False {
            }
            frame True {
              n191 = call "Server_Emails.vi"("Client Name Contains"="EnFlo_Tunnel", "Message"="The pressure in the chilled water  for the Enflo Tunnel has tripped the system. The chiller pumps should automaticaly be turned off and the cooling circuit isolated from the  University Chilled water system. The heaters should also have been disabled.", "Subject"="EnFlo Chilled Water Overpressure Trip") -> ()  [unwired: 2 in, 3 out]
            }
          }
          n192 = call "Running_Ch_Average.vi"("Shift In"=w439, "History length"=65, "New Value"=w432) -> ("Shift Out"=w440:dbl[], "mean"=w437:dbl)  [unwired: 2 in, 1 out]
          n193 = Concatenate Strings(w431, w449, w450) -> (w448:string)
        }
      }
      frame #12 {
        n194 = Compound Arithmetic op=AND(w462, w464, w463) -> (w465:bool)
        n195 = case shown="False" w465 {
          tunnel: w468 -> [w473 _]
          tunnel: w467 -> [w472 _]
          tunnel: [w469 ""] -> w466
          frame False {
            n196 = for {
              tunnel: w473 -> [w483]
              tunnel: w472 -> [w482]
              tunnel: string[] ["EnFlo_Tunnel:Heater:Enable"] ("Ch Names") -> [w478] mode=indexing
              shift-right: [w476] -> w469
              shift-left: "" -> [w477]
              n197 = call "Read_value_of_earlier_Ch.vi"("Desired Ch to Read"=w478, "Ch names"=w482, "Present scan array"=w483) -> ("Value"=w480:dbl, "Scan comment"=w475:string)  [unwired: 1 in]
              n198 = Greater?(x=w480, y=0.5) -> (0:w479:bool)
              n199 = case shown="True" w479 {
                tunnel: w478 -> [_ w488]
                tunnel: ["" w485] -> w474
                frame False {
                }
                frame True {
                  n200 = Build Array(w488) -> (w491:string[])
                  n201 = Build Array(0.0) -> (w490:dbl[])
                  n202 = call "ASYNC_Adam_server.vi"("Values"=w490, "Channel Names"=w491) -> ("Scan Comments"=w486:string[])  [unwired: 1 in, 2 out]
                  n203 = Index Array(array=w486, index=0) -> (element=w485:string)
                }
              }
              n204 = Concatenate Strings(w477, w475, w474) -> (w476:string)
            }
          }
          frame True {
          }
        }
      }
      frame #13 {
        n205 = case shown="False" w493 {
          tunnel: w496 -> [w501 _]
          tunnel: w495 -> [w500 _]
          tunnel: [w506 ""] -> w494
          frame False {
            w499 = "EnFlo_Tunnel:Tap_Water:Enable" ("Ch Name")
            n206 = call "Read_value_of_earlier_Ch.vi"("Desired Ch to Read"=w499, "Ch names"=w500, "Present scan array"=w501) -> ("Value"=w504:dbl, "Scan comment"=w498:string)  [unwired: 1 in]
            n207 = Greater?(x=w504, y=0.5) -> (0:w502:bool)
            n208 = case shown="True" w502 {
              tunnel: [w507 w516] -> w503
              tunnel: w501 -> [_ w515]
              tunnel: w500 -> [_ w514]
              tunnel: w499 -> [_ w509]
              tunnel: [w507 w508] -> w497
              frame False {
                w507 = ""
              }
              frame True {
                n209 = call "Read_value_of_earlier_Ch.vi"("Desired Ch to Read"="EnFlo_Tunnel:Inlet_Temp:Average" ("Ch Name"), "Ch names"=w514, "Present scan array"=w515) -> ("Value"=w512:dbl, "Scan comment"=w508:string)  [unwired: 1 in]
                n210 = Less?(x=w512, y=30.0) -> (x < y?=w510:bool)
                n211 = case shown="True" w510 {
                  tunnel: w509 -> [_ w521]
                  tunnel: ["" w518] -> w516
                  frame False {
                  }
                  frame True {
                    n212 = Build Array(w521) -> (w524:string[])
                    n213 = Build Array(0.0) -> (w523:dbl[])
                    n214 = call "ASYNC_Adam_server.vi"("Values"=w523, "Channel Names"=w524) -> ("Scan Comments"=w519:string[])  [unwired: 1 in, 2 out]
                    n215 = Index Array(array=w519, index=0) -> (element=w518:string)
                  }
                }
              }
            }
            n216 = Concatenate Strings(w498, w497, w503) -> (w506:string)
          }
          frame True {
          }
        }
      }
      frame #14 {
        n217 = while {
          tunnel: w528 -> [w544]
          tunnel: w527 -> [w543]
          shift-right: [w537] -> _
          shift-left: _ -> [w533]
          tunnel: [w529] -> w526
          stop <- FALSE continue-if-true
          w535 = 60.0 ("y")
          n218 = Decrement(x=w535) -> (x-1=w536:dbl)
          n219 = Select(t=w536, s=w533, f=w535) -> (s? t:f=w534:dbl)
          n220 = call "Read_value_of_earlier_Ch.vi"("Desired Ch to Read"="EnFlo_Tunnel:Chilled Water:Motor1 Temp", "Ch names"=w543, "Present scan array"=w544) -> ("Value"=w551:dbl, "Scan comment"=w531:string)  [unwired: 1 in]
          n221 = call "Read_value_of_earlier_Ch.vi"("Desired Ch to Read"="EnFlo_Tunnel:Chilled Water:Motor2 Temp", "Ch names"=w543, "Present scan array"=w544) -> ("Value"=w548:dbl, "Scan comment"=w530:string)  [unwired: 1 in]
          n222 = Greater?(x=w551, y=w534) -> (0:w545:bool)
          n223 = Greater?(x=w548, y=w534) -> (0:w546:bool)
          n224 = Or(x=w545, y=w546) -> (x .or. y?=w539:bool)
          n225 = call "Read_value_of_earlier_Ch.vi"("Desired Ch to Read"="EnFlo_Tunnel:Chiller_Pump:Running", "Ch names"=w543, "Present scan array"=w544) -> ("Value"=w541:dbl, "Scan comment"=w532:string)  [unwired: 1 in]
          n226 = Greater?(x=w541, y=0.5) -> (0:w538:bool)
          n227 = And(x=w538, y=w539) -> (x .and. y?=w537:bool)
          n228 = Compound Arithmetic op=AND(w537, invert w533) -> (w550:bool)
          n229 = case shown="True" w550 {
            tunnel: w535 -> [_ w554]
            frame False {
            }
            frame True {
              n230 = Format Into String(format string="The Chilled Water Motor Temp is greater than %.0f deg C." ("Message"), w554) -> (resulting string=w553:string)  [unwired: 2 in, 1 out]
              n231 = call "Server_Emails.vi"("Client Name Contains"="EnFlo_Tunnel", "Message"=w553, "Subject"="Chilled Water Motor Temp") -> ()  [unwired: 2 in, 3 out]
            }
          }
          n232 = Concatenate Strings(w532, w531, w530) -> (w529:string)
        }
      }
      frame #15 {
        n233 = while {
          tunnel: w562 -> [w591]
          tunnel: w561 -> [w590]
          shift-right: [w589] -> _
          shift-left: _ -> [w588]
          tunnel: [w585] -> w560
          shift-right: [w578] -> _
          shift-left: _ -> [w579]
          tunnel: w559 -> [w573]
          tunnel: w558 -> [w563]
          stop <- FALSE continue-if-true
          w582 = "EnFlo_Lab:Ozone:(ppb)" ("Desired Ch to Read")
          w576 = "EnFlo_Tunnel:Ozone_Generators:Enable" ("Desired Ch to Read")
          n234 = case shown="7..19" w573 {
            tunnel: [w597 w600] -> w566
            tunnel: [w596 w598] -> w572
            frame Default {
              w597 = 200.0
              n235 = Format Into String(format string=" The night time limit has been set as %.0fppb over 15 minutes.", w597) -> (resulting string=w596:string)  [unwired: 2 in, 1 out]
            }
            frame 7..19 {
              w600 = 60.0
              n236 = Format Into String(format string=" The day time limit has been set as %.0fppb over 15 minutes.", w600) -> (resulting string=w598:string)  [unwired: 2 in, 1 out]
            }
          }
          n237 = call "Read_value_of_earlier_Ch.vi"("Desired Ch to Read"=w576, "Ch names"=w590, "Present scan array"=w591) -> ("Value"=w594:dbl, "Scan comment"=w586:string)  [unwired: 1 in]
          n238 = Greater?(x=w594, y=0.5) -> (0:w583:bool)
          n239 = call "Read_value_of_earlier_Ch.vi"("Desired Ch to Read"=w582, "Ch names"=w590, "Present scan array"=w591) -> ("Value"=w581:dbl, "Scan comment"=w587:string)  [unwired: 1 in]
          n240 = call "Running_Ch_Average.vi"("Shift In"=w579, "History length"=450, "Reset Average after Seconds"=120.0, "New Value"=w581) -> ("Shift Out"=w578:dbl[], "standard deviation"=w570:dbl, "mean"=w577:dbl)  [unwired: 1 in]
          n241 = Add(x=4.0, y=w566) -> (x+y=w565:dbl)
          n242 = Greater?(x=w577, y=w565) -> (0:w571:bool)
          n243 = Less?(x=w570, y="Minimum St Dev for Ozone inst") -> (x < y?=w568:bool)
          n244 = Or(x=w571, y=w568) -> (x .or. y?=w567:bool)
          n245 = And(x=w567, y=w583) -> (x .and. y?=w589:bool)
          n246 = Compound Arithmetic op=AND(w589, invert w588, w563) -> (w593:bool)
          n247 = case shown="True" w593 {
            tunnel: w577 -> [_ w610]
            tunnel: w582 -> [_ w608]
            tunnel: w576 -> [_ w607]
            tunnel: ["" w603] -> w575
            tunnel: w572 -> [_ w602]
            frame False {
            }
            frame True {
              n248 = Build Array(w607) -> (w606:string[])
              n249 = call "ASYNC_Adam_server.vi"("Values"=dbl[] [0.0], "Channel Names"=w606) -> ("Scan Comments"=w604:string[])  [unwired: 1 in, 2 out]
              n250 = Format Into String(format string="The %s is greater than %.0f ppb.%s" ("Message"), w608, w610, w602) -> (resulting string=w609:string)  [unwired: 2 in, 1 out]
              n251 = call "Server_Emails.vi"("Client Name Contains"="EnFlo_Tunnel", "Message"=w609, "Subject"="Ozone level Warning") -> ()  [unwired: 2 in, 3 out]
              n252 = Concatenate Strings(w604) -> (w603:string)
            }
          }
          n253 = Concatenate Strings(w587, w586, w575) -> (w585:string)
        }
      }
      frame #16 {
        n254 = call "Read_value_of_earlier_Ch.vi"("Desired Ch to Read"="EnFlo_Tunnel:FFID:Enable", "Ch names"=w634, "Present scan array"=w635) -> ("Value"=w629:dbl, "Scan comment"=w615:string)  [unwired: 1 in]
        n255 = call "Read_value_of_earlier_Ch.vi"("Desired Ch to Read"="Aero_Tunnel:FFID:Enable", "Ch names"=w634, "Present scan array"=w635) -> ("Value"=w630:dbl, "Scan comment"=w616:string)  [unwired: 1 in]
        n256 = call "Read_value_of_earlier_Ch.vi"("Desired Ch to Read"="A_Tunnel:FFID:Enable", "Ch names"=w634, "Present scan array"=w635) -> ("Value"=w625:dbl, "Scan comment"=w617:string)  [unwired: 1 in]
        n257 = call "Read_value_of_earlier_Ch.vi"("Desired Ch to Read"="GMU:Gas:Enable", "Ch names"=w634, "Present scan array"=w635) -> ("Value"=w623:dbl, "Scan comment"=w618:string)  [unwired: 1 in]
        n258 = Concatenate Strings(w618, w617, w616, w615) -> (w614:string)
        n259 = Build Array(w625, w630, w629) -> (w628:dbl[])
        n260 = Greater?(x=w623, y=0.5) -> (0:w619:bool)
        n261 = Greater?(x=w628, y=0.5) -> (0:w627:bool[])
        n262 = Or Array Elements(Boolean array=w627) -> (logical OR=w621:bool)
        n263 = Equal?(x=w619, y=w621) -> (x = y?=w620:bool)
        n264 = case shown="False" w620 {
          tunnel: w619 -> [w637 _]
          frame False {
            n265 = Not(x=w637) -> (.not. x?=w636:bool)
            n266 = Select(t=1.0, s=w636, f=0.0 ("t")) -> (s? t:f=w640:dbl)
            n267 = Build Array(w640) -> (w642:dbl[])
            n268 = call "ASYNC_Adam_server.vi"("Values"=w642, "Channel Names"=string[] ["GMU:Gas:Enable"]) -> ()  [unwired: 1 in, 3 out]
          }
          frame True {
          }
        }
      }
      frame #17 {
        n269 = while {
          tunnel: w647 -> [w659]
          tunnel: w646 -> [w658]
          shift-right: [w649] -> _
          shift-left: _ -> [w654]
          tunnel: [w653] -> w645
          tunnel: w644 -> [w651]
          tunnel: w643 -> [w648]
          stop <- FALSE continue-if-true
          w650 = "EnFlo_Tunnel:Motor:Enable" ("Desired Ch to Read")
          # "Re Zero EnFlo Tunnel static pressure when turning tunnel on"
          n270 = call "Read_value_of_earlier_Ch.vi"("Desired Ch to Read"=w650, "Ch names"=w658, "Present scan array"=w659) -> ("Value"=w655:dbl, "Scan comment"=w653:string)  [unwired: 1 in]
          n271 = Greater?(x=w655, y=0.5) -> (0:w649:bool)
          n272 = Compound Arithmetic op=AND(w649, invert w654, w648) -> (w652:bool)
          n273 = case shown="True" w652 {
            tunnel: w651 -> [_ w682]
            tunnel: w650 -> [_ w680]
            frame False {
            }
            frame True {
              w679 = "EnFlo_Tunnel:Pressure:Static"
              n274 = Build Array(w679) -> (w678:string[])
              n275 = Build Array(w680, w679) -> (w683:string[])
              n276 = Subtract(x=w682, y=15.0) -> (x-y=w668:dbl)
              n277 = call "Get_Current_Scan_server.vi"("Desired Channels"=w678) -> ("Ch Description Array"=w677:T9[])  [unwired: 2 out]
              n278 = Subtract(x=w682, y=3600.0) -> (x-y=w681:dbl)
              n279 = call "Get_ADAM_averages_server.vi"("No of averages"=600, "End time"=w668, "Start time"=w681, "Clients time"=w682, "ADAM Ch Names"=w683) -> ("DBL values"=w671:dbl[][])  [unwired: 1 in, 4 out]
              n280 = Index Array(array=w677) -> (element=w675:T9)  [unwired: 1 in]
              n281 = Unbundle By Name(w675) -> ("A"=w676:dbl)
              n282 = Index Array(array=w671, index (col)=1 ("disabled index (col)")) -> (element=w667:dbl[])  [unwired: 1 in]
              n283 = Index Array(array=w671, index (col)=2 ("disabled index (col)")) -> (element=w666:dbl[])  [unwired: 1 in]
              n284 = Reverse 1D Array(array=w666) -> (reversed array=w662:dbl[])
              n285 = Reverse 1D Array(array=w667) -> (reversed array=w665:dbl[])
              n286 = for {
                tunnel: w665 -> [w690] mode=indexing
                tunnel: [w689] -> w664 mode=indexing
                tunnel: w662 -> [w689] mode=indexing
                stop <- w691 continue-if-true
                n287 = Less?(x=w690, y=0.01) -> (x < y?=w691:bool)
              }
              n288 = call "Mean_fr_NaN_data.vi"("Data"=w664) -> ("Mean value"=w663:dbl)  [unwired: 1 out]
              n289 = Subtract(x=w676, y=w663) -> (x-y=w661:dbl)
              n290 = Not A Number/Path/Refnum?(number/path/refnum=w661) -> (NaN/Path/Refnum?=w660:bool)
              n291 = case shown="True" w660 {
                tunnel: w675 -> [w688 _]
                tunnel: w661 -> [w687 _]
                frame False {
                  n292 = Bundle By Name(cluster=w688, "A"=w687) -> (w686:T9)
                  n293 = Build Array(w686) -> (w685:T9[])
                  n294 = call "Update_Ch_Discription_server.vi"("Mode"=T2."Append to Global", "Channels to update In"=w685) -> ()  [unwired: 1 in, 1 out]
                }
                frame True {
                }
              }
            }
          }
        }
      }
      frame #18 {
        # "Resetting A Tunnel speed to zero if the drive in turned off\nso that the belts do not slip when the tunnel is turned on again."
        n295 = while {
          tunnel: w696 -> [w709]
          tunnel: w695 -> [w708]
          shift-right: [w700] -> _
          shift-left: _ -> [w703]
          shift-left: _ -> [w702]
          shift-left: _ -> [w701]
          tunnel: w694 -> [w699]
          tunnel: [w697] -> w693
          stop <- FALSE continue-if-true
          n296 = call "Read_value_of_earlier_Ch.vi"("Desired Ch to Read"="A_Tunnel:Motor:Enable", "Ch names"=w708, "Present scan array"=w709) -> ("Value"=w704:dbl, "Scan comment"=w697:string)  [unwired: 1 in]
          n297 = Less?(x=w704, y=0.5) -> (x < y?=w700:bool)
          n298 = Compound Arithmetic op=AND(w700, w703, invert w702, invert w701, w699) -> (w698:bool)
          n299 = case shown="True" w698 {
            tunnel: w700 -> [_ _]
            frame False {
            }
            frame True {
              w712 = string[] ["A_Tunnel:Speed:Dem Velocity", "A_Tunnel:Speed:Dem Voltage"] ("Channel Names")
              n300 = Array Size(array=w712) -> (size(s)=w713:i32)
              n301 = Initialize Array(0.0 ("element"), w713) -> (w711:dbl[])
              n302 = call "ASYNC_Adam_server.vi"("Values"=w711, "Channel Names"=w712) -> ()  [unwired: 1 in, 3 out]
            }
          }
        }
      }
      frame #19 {
        n303 = global read "EnFlo_Tunnel_Global.vi" "Minimum Shaft RPM"() -> (w719:dbl)
        n304 = call "Read_value_of_earlier_Ch.vi"("Desired Ch to Read"="EnFlo_Tunnel:Motor 1:RPM", "Ch names"=w717, "Present scan array"=w718) -> ("Value"=w716:dbl)  [unwired: 1 in, 1 out]
        n305 = Greater?(x=w716, y=w719) -> (0:w715:bool)
      }
      frame #20 {
        # "Control Inlet fans"
        n306 = while {
          tunnel: w722 -> [w728]
          tunnel: w721 -> [w726]
          shift-right: [w725] -> _
          shift-left: _ -> [w731]
          tunnel: [w724] -> w720
          stop <- FALSE continue-if-true
          n307 = call "Read_value_of_earlier_Ch.vi"("Desired Ch to Read"="EnFlo_Tunnel:Motor:Enable", "Ch names"=w726, "Present scan array"=w728) -> ("Value"=w727:dbl, "Scan comment"=w724:string)  [unwired: 1 in]
          n308 = Greater?(x=w727, y=0.5) -> (0:w725:bool)
          n309 = Not Equal?(x=w725, y=w731) -> (x != y?=w730:bool)
          n310 = Compound Arithmetic op=AND(invert w725, w730) -> (w732:bool)
          n311 = case shown="True" w732 {
            tunnel: w725 -> [_ _]
            tunnel: w726 -> [_ w737]
            frame False {
            }
            frame True {
              w738 = "EnFlo_Tunnel:Power:Inlet Fan"
              n312 = String Length(string=w738) -> (length=w739:i32)
              n313 = for {
                tunnel: w737 -> [w744] mode=indexing
                tunnel: w739 -> [w747]
                tunnel: w738 -> [w746]
                tunnel: [w744] -> w735 mode=indexing if=w743
                n314 = String Subset(string=w744, length (rest)=w747) -> (substring=w745:string)  [unwired: 1 out]
                n315 = Equal?(x=w745, y=w746) -> (x = y?=w743:bool)
              }
              n316 = Build Array (concatenate)(string[] ["EnFlo_Tunnel:Trav_Blockage_Fans:Dem_Volts"] ("Channel Names"), w735) -> (w734:string[])
              n317 = Array Size(array=w734) -> (size(s)=w742:i32)
              n318 = Initialize Array(0.0 ("element"), w742) -> (w741:dbl[])
              n319 = call "ASYNC_Adam_server.vi"("Values"=w741, "Channel Names"=w734) -> ()  [unwired: 1 in, 3 out]
            }
          }
        }
      }
      frame #21 {
        # "EnFlo_Tunnel:Inlet_Temp:Average - Uni:Chilled Water:Temp"
        n320 = call "Read_Earlier_Channels.vi"("Present scan array"=w751, "Ch names"=w750, "Desired Channels"=string[] ["EnFlo_Tunnel:Inlet_Temp:Average", "Uni:Chilled Water:Temp"]) -> ("Scan comments"=w748:string, "Index 0"=w753:dbl, "Index 1"=w752:dbl)  [unwired: 3 out]
        n321 = Subtract(x=w753, y=w752) -> (x-y=w749:dbl)
      }
      frame #22 {
        n322 = case shown="True" w759 {
          selector: w759 -> [w760 _]
          tunnel: w758 -> [_ w765]
          tunnel: w757 -> [_ w763]
          tunnel: w756 -> [_ w762]
          tunnel: [w760 w761] -> w755
          frame False {
          }
          frame True {
            n323 = Greater Than 0?(x=w765) -> (x > 0?=w764:bool)
            n324 = case shown="True" w764 {
              tunnel: w763 -> [_ w770]
              tunnel: w762 -> [_ w769]
              tunnel: [TRUE w767] -> w761
              frame False {
              }
              frame True {
                n325 = for {
                  tunnel: w770 -> [w776]
                  tunnel: w769 -> [w775]
                  tunnel: string[] ["EnFlo_Tunnel:Power:Exit_Heaters", "EnFlo_Lab:Fan_Heater_1:Enable", "EnFlo_Lab:Fan_Heater_2:Enable"] -> [w774] mode=indexing
                  tunnel: [w771] -> w767
                  stop <- w771 continue-if-true
                  n326 = call "Read_value_of_earlier_Ch.vi"("Desired Ch to Read"=w774, "Ch names"=w775, "Present scan array"=w776) -> ("Value"=w773:dbl)  [unwired: 1 in, 1 out]
                  n327 = Less?(x=w773, y=0.5) -> (x < y?=w771:bool)
                }
              }
            }
          }
        }
      }
      frame #23 {
        n328 = case shown="True" w778 {
          tunnel: w783 -> [_ w800]
          tunnel: w782 -> [_ w799]
          tunnel: [0.0 ("upper limit") w801] -> w781
          tunnel: ["" w796] -> w780
          tunnel: w779 -> [_ w797]
          tunnel: w777 -> [_ w786]
          frame False {
          }
          frame True {
            n329 = Greater Than 0?(x=w797) -> (x > 0?=w798:bool)
            n330 = call "Read_Earlier_Channels.vi"("Present scan array"=w800, "Ch names"=w799, "Desired Channels"=string[] ["EnFlo_Tunnel:Exit Duct:Dem Temp", "EnFlo_Tunnel:Heat_Ex_Div_Valve:Dem Pos", "EnFlo_Tunnel:Exit Duct Temp:Average"] ("appended array")) -> ("Scan comments"=w796:string, "Index 0"=w790:dbl, "Index 1"=w792:dbl, "Index 2"=w788:dbl)  [unwired: 2 out]
            n331 = case shown="False" w798 {
              tunnel: w790 -> [w803 w805]
              tunnel: [w802 w805] -> w789
              tunnel: w788 -> [w802 w804]
              tunnel: [w803 w804] -> w787
              frame False {
              }
              frame True {
              }
            }
            n332 = call "Back_End_Chiller_PID.vi"("Setpoint"=w789, "Current Time"=w786, "Previous Control Sum"=w792, "Present Value"=w787) -> ("Dem Output"=w795:dbl)  [unwired: 1 in]
            n333 = In Range and Coerce(upper limit=100.0, x=w795, lower limit=0.0) -> (coerced(x)=w801:dbl)  [unwired: 1 out]
          }
        }
      }
      frame #24 {
        n334 = feedback #5() -> (w812:dbl[])  [unwired: 1 in]
        n335 = call "Running_Ch_Average.vi"("Shift In"=w812, "History length"=600, "Reset Average after Seconds"=100.0, "New Value"=w808) -> ("Shift Out"=w809:dbl[], "mean"=w807:dbl)  [unwired: 1 in, 1 out]
        n336 = feedback-in #5(w809) -> ()
        n337 = case shown="True" w816 {
          tunnel: w819 -> [_ w831]
          tunnel: w818 -> [_ w830]
          tunnel: [FALSE w843] -> w817
          tunnel: w808 -> [_ _]
          tunnel: ["" w824] -> w815
          tunnel: [FALSE w840] -> w814
          tunnel: w813 -> [_ w838]
          tunnel: w807 -> [_ w834]
          tunnel: w806 -> [_ w833]
          frame False {
          }
          frame True {
            n338 = call "Read_value_of_earlier_Ch.vi"("Desired Ch to Read"="EnFlo Lab:Leak_Detector_Circuit:Happy", "Ch names"=w830, "Present scan array"=w831) -> ("Value"=w827:dbl, "Scan comment"=w825:string)  [unwired: 1 in]
            n339 = Greater Than 0?(x=w833) -> (x > 0?=w842:bool)
            n340 = Greater?(x=w827, y=0.5) -> (0:w823:bool)
            n341 = Select(t=0.05 ("y"), s=w838, f=0.6 ("t")) -> (s? t:f=w837:dbl)
            n342 = call "Read_Earlier_Channels.vi"("Present scan array"=w831, "Ch names"=w830, "Desired Channels"=string[] ["EnFlo Lab:Emergency_Stop:Happy", "EnFlo Lab:Leak_Detector:Happy", "EnFlo_Tunnel:Floor_Cooling:Enable", "EnFlo Lab:Heat:Extraction"]) -> ("Scan comments"=w826:string, "Index 0"=w846:dbl, "Index 1"=w845:dbl, "Index 2"=w844:dbl, "Index 3"=w832:dbl)  [unwired: 1 out]
            n343 = case shown="False" w842 {
              tunnel: w833 -> [w862 w870]
              tunnel: [w859 w869] -> w841
              tunnel: w832 -> [w863 _]
              tunnel: [w859 FALSE] -> w840
              tunnel: w838 -> [w857 w867]
              frame False {
                n344 = Select(t=-0.2 ("y"), s=w857, f=-0.8 ("y")) -> (s? t:f=w858:dbl)
                n345 = Less Than 0?(x=w863) -> (x < 0?=w860:bool)
                n346 = Less?(x=w862, y=w858) -> (x < y?=w861:bool)
                n347 = And(x=w861, y=w860) -> (x .and. y?=w859:bool)
              }
              frame True {
                n348 = Select(t=0.0 ("y"), s=w867, f=1.0 ("y")) -> (s? t:f=w865:dbl)
                n349 = Greater?(x=w870, y=w865) -> (0:w869:bool)
              }
            }
            n350 = Concatenate Strings(w825, w826) -> (w824:string)
            n351 = Greater?(x=w834, y=w837) -> (0:w839:bool)
            n352 = Greater?(x=w846, y=0.5) -> (0:w848:bool)
            n353 = Greater?(x=w845, y=0.5) -> (0:w849:bool)
            n354 = Greater?(x=w844, y=0.5) -> (0:w853:bool)
            n355 = Or(x=w853, y=w839) -> (x .or. y?=w850:bool)
            n356 = Compound Arithmetic op=AND(w823, w841, w848, w849, w850) -> (w843:bool)
          }
        }
      }
      frame #25 {
        n357 = case shown="True" w873 {
          tunnel: w872 -> [_ w878]
          tunnel: ["" w875] -> w871
          frame False {
          }
          frame True {
            n358 = Greater?(x=w878, y=-0.35) -> (0:w876:bool)
            n359 = case shown="True" w876 {
              tunnel: ["" w880] -> w875
              frame False {
              }
              frame True {
                n360 = Build Array("EnFlo_Tunnel:Chiller_Pump:Enable" ("Desired Ch to Read"), "EnFlo_Tunnel:Chilled Water:Motor_Dem_Voltage" ("Desired Ch to Read"), "EnFlo_Tunnel:Chiller_Pump_Drive:Enable" ("Desired Ch to Read")) -> (w887:string[])
                n361 = for {
                  tunnel: [w889] -> w883 mode=indexing
                  tunnel: w887 -> [w889] mode=indexing
                  tunnel: [0.0] -> w886 mode=indexing
                }
                n362 = call "ASYNC_Adam_server.vi"("Values"=w886, "Channel Names"=w883) -> ("Scan Comments"=w882:string[])  [unwired: 1 in, 2 out]
                n363 = Concatenate Strings(w882) -> (w880:string)
              }
            }
          }
        }
      }
      frame #26 {
        n364 = case shown="True" w895 {
          tunnel: w897 -> [w908 w930]
          tunnel: w896 -> [w907 w929]
          tunnel: [w898 w927] -> w894
          tunnel: [w899 w923] -> w893
          tunnel: w892 -> [_ w922]
          tunnel: [w909 0] -> w891
          tunnel: w890 -> [w904 _]
          frame False {
            w900 = "EnFlo_Tunnel:Chiller_Pump:Enable" ("Desired Ch to Read")
            n365 = call "Read_value_of_earlier_Ch.vi"("Desired Ch to Read"=w900, "Ch names"=w907, "Present scan array"=w908) -> ("Value"=w906:dbl)  [unwired: 1 in, 1 out]
            n366 = Greater?(x=w906, y=0.5) -> (0:w898:bool)
            n367 = Greater?(x=w904, y=100) -> (0:w902:bool)
            n368 = And(x=w902, y=w898) -> (x .and. y?=w901:bool)
            n369 = case shown="True" w901 {
              tunnel: w900 -> [_ w914]
              tunnel: ["" w911] -> w899
              frame False {
              }
              frame True {
                n370 = Build Array(w914, "EnFlo_Tunnel:Chilled Water:Motor_Dem_Voltage" ("Desired Ch to Read"), "EnFlo_Tunnel:Chiller_Pump_Drive:Enable" ("Desired Ch to Read")) -> (w918:string[])
                n371 = for {
                  tunnel: [w920] -> w913 mode=indexing
                  tunnel: w918 -> [w920] mode=indexing
                  tunnel: [0.0] -> w917 mode=indexing
                }
                n372 = call "ASYNC_Adam_server.vi"("Values"=w917, "Channel Names"=w913) -> ("Scan Comments"=w912:string[])  [unwired: 1 in, 2 out]
                n373 = Concatenate Strings(w912) -> (w911:string)
              }
            }
            n374 = Increment(x=w904) -> (x+1=w909:i32)
          }
          frame True {
            w933 = "EnFlo_Tunnel:Chiller_Pump:Enable"
            n375 = Greater?(x=w922, y=0.99) -> (0:w928:bool)
            n376 = case shown="True" w928 {
              tunnel: w930 -> [_ w946]
              tunnel: w929 -> [_ w945]
              tunnel: [FALSE w944] -> w927
              tunnel: ["" w943] -> w924
              frame False {
              }
              frame True {
                w941 = "EnFlo_Tunnel:Chiller_Pump_Drive:Enable"
                n377 = call "Read_value_of_earlier_Ch.vi"("Desired Ch to Read"=w941, "Ch names"=w945, "Present scan array"=w946) -> ("Value"=w942:dbl, "Scan comment"=w938:string)  [unwired: 1 in]
                n378 = Greater?(x=w942, y=0.5) -> (0:w940:bool)
                n379 = case shown="True" w940 {
                  tunnel: w941 -> [w954 _]
                  tunnel: [FALSE TRUE] -> w944
                  tunnel: w938 -> [w948 w955]
                  tunnel: [w947 w955] -> w943
                  frame False {
                    n380 = Build Array(1.0 ("y")) -> (w952:dbl[])
                    n381 = Build Array(w954) -> (w953:string[])
                    n382 = call "ASYNC_Adam_server.vi"("Values"=w952, "Channel Names"=w953) -> ("Scan Comments"=w949:string[])  [unwired: 1 in, 2 out]
                    n383 = Concatenate Strings(w948, w949) -> (w947:string)
                  }
                  frame True {
                  }
                }
              }
            }
            n384 = call "Read_value_of_earlier_Ch.vi"("Desired Ch to Read"=w933, "Ch names"=w929, "Present scan array"=w930) -> ("Value"=w932:dbl, "Scan comment"=w926:string)  [unwired: 1 in]
            n385 = Greater?(x=w932, y=0.5) -> (0:w934:bool)
            n386 = case shown="False" w934 {
              tunnel: w933 -> [w961 _]
              tunnel: [w957 string[] [] ("Scan Comments")] -> w925
              frame False {
                n387 = Build Array(1.0 ("y")) -> (w959:dbl[])
                n388 = Build Array(w961) -> (w960:string[])
                n389 = call "ASYNC_Adam_server.vi"("Values"=w959, "Channel Names"=w960) -> ("Scan Comments"=w957:string[])  [unwired: 1 in, 2 out]
              }
              frame True {
              }
            }
            n390 = Concatenate Strings(w926, w925, w924) -> (w923:string)
          }
        }
      }
      frame #27 {
        n391 = case shown="True" w964 {
          tunnel: w969 -> [w975 w1005]
          tunnel: w968 -> [w974 w1004]
          tunnel: [w970 w998] -> w967
          tunnel: [TRUE w990] -> w966
          tunnel: [0.0 ("Value") w992] -> w965
          tunnel: w963 -> [_ w991]
          frame False {
            w973 = 0.0 ("lower limit")
            w978 = "EnFlo_Tunnel:Chilled Water:Motor_Dem_Voltage"
            n392 = call "Read_value_of_earlier_Ch.vi"("Desired Ch to Read"=w978, "Ch names"=w974, "Present scan array"=w975) -> ("Value"=w976:dbl, "Scan comment"=w971:string)  [unwired: 1 in]
            n393 = Equal?(x=w976, y=w973) -> (x = y?=w977:bool)
            n394 = case shown="False" w977 {
              tunnel: w978 -> [w983 _]
              tunnel: w973 -> [w982 _]
              tunnel: [w981 string[] [] ("Scan Comments")] -> w972
              frame False {
                n395 = Build Array(w983) -> (w984:string[])
                n396 = Build Array(w982) -> (w985:dbl[])
                n397 = call "ASYNC_Adam_server.vi"("Values"=w985, "Channel Names"=w984) -> ("Scan Comments"=w981:string[])  [unwired: 1 in, 2 out]
              }
              frame True {
              }
            }
            n398 = Concatenate Strings(w971, w972) -> (w970:string)
          }
          frame True {
            w1001 = "EnFlo_Tunnel:Chilled Water:Motor_Dem_Voltage"
            # "EnFlo_Tunnel:Chiller_Pump:Running"
            n399 = call "Read_value_of_earlier_Ch.vi"("Desired Ch to Read"="EnFlo_Tunnel:Chilled Water:Pressure_supply (Bar)", "Ch names"=w1004, "Present scan array"=w1005) -> ("Value"=w997:dbl, "Scan comment"=w1000:string)  [unwired: 1 in]
            n400 = call "Read_value_of_earlier_Ch.vi"("Desired Ch to Read"=w1001, "Ch names"=w1004, "Present scan array"=w1005) -> ("Value"=w992:dbl, "Scan comment"=w999:string)  [unwired: 1 in]
            n401 = Concatenate Strings(w1000, w999) -> (w998:string)
            n402 = Less?(x=w997, y=3.95) -> (x < y?=w990:bool)
            n403 = case shown="True" w990 {
              tunnel: w992 -> [w1008 w1011]
              tunnel: [w1007 w1010] -> w988
              tunnel: w991 -> [_ _]
              frame False {
                n404 = Subtract(x=w1008, y=0.1) -> (x-y=w1007:dbl)
              }
              frame True {
                n405 = Equal To 0?(x=w1011) -> (x = 0?=w1012:bool)
                n406 = Select(t=5.9, s=w1012, f=w1011) -> (s? t:f=w1010:dbl)
              }
            }
            n407 = Select(t=0.0, s=w990, f=w988) -> (s? t:f=w989:dbl)
            n408 = In Range and Coerce(upper limit=10.0, x=w989, lower limit=0.0) -> (coerced(x)=w993:dbl)  [unwired: 1 out]
            n409 = Equal?(x=w992, y=w993) -> (x = y?=w996:bool)
            n410 = case shown="False" w996 {
              tunnel: w1001 -> [w1014 _]
              tunnel: w993 -> [w1013 _]
              frame False {
                n411 = Build Array(w1014) -> (w1015:string[])
                n412 = Build Array(w1013) -> (w1016:dbl[])
                n413 = call "ASYNC_Adam_server.vi"("Values"=w1016, "Channel Names"=w1015) -> ()  [unwired: 1 in, 3 out]
              }
              frame True {
              }
            }
          }
        }
      }
      frame #28 {
        w1020 = "EnFlo lab:Using Chilled Water:To Heat"
        n414 = And(x=w1029, y=w1028) -> (x .and. y?=w1025:bool)
        n415 = Select(t=1.0, s=w1025, f=0.0) -> (s? t:f=w1019:dbl)
        n416 = call "Read_value_of_earlier_Ch.vi"("Desired Ch to Read"=w1020, "Ch names"=w1026, "Present scan array"=w1027) -> ("Value"=w1022:dbl, "Scan comment"=w1018:string)  [unwired: 1 in]
        n417 = Equal?(x=w1022, y=w1019) -> (x = y?=w1021:bool)
        n418 = case shown="False" w1021 {
          tunnel: w1020 -> [w1034 _]
          tunnel: w1019 -> [w1033 _]
          tunnel: w1018 -> [w1032 w1037]
          tunnel: [w1030 w1037] -> w1017
          frame False {
            n419 = Build Array(w1034) -> (w1035:string[])
            n420 = Build Array(w1033) -> (w1036:dbl[])
            n421 = call "ASYNC_Adam_server.vi"("Values"=w1036, "Channel Names"=w1035) -> ("Scan Comments"=w1031:string[])  [unwired: 1 in, 2 out]
            n422 = Concatenate Strings(w1032, w1031) -> (w1030:string)
          }
          frame True {
          }
        }
      }
      frame #29 {
        n423 = Or(x=w1039, y=w1040) -> (x .or. y?=w1038:bool)
        n424 = case shown="True" w1038 {
          tunnel: [w1049 w1060] -> w1046
          tunnel: w1042 -> [_ w1060]
          tunnel: [w1048 FALSE] -> w1044
          frame False {
            # "Exercise valve once a week"
            n425 = Seconds To Date/Time() -> (date time rec=w1050:T8)  [unwired: 2 out]
            n426 = Unbundle By Name(w1050) -> ("day of week"=w1055:i32, "hour"=w1053:i32)
            n427 = Less?(x=w1053, y=3) -> (x < y?=w1058:bool)
            n428 = Equal?(x=7, y=w1055) -> (x = y?=w1057:bool)
            n429 = And(x=w1057, y=w1058) -> (x .and. y?=w1048:bool)
            n430 = Select(t=100.0, s=w1048, f=0.0) -> (s? t:f=w1049:dbl)
          }
          frame True {
          }
        }
        n431 = while {
          shift-right: [w1066] -> _
          shift-left: _ -> [w1067]
          tunnel: w1046 -> [w1066]
          tunnel: "EnFlo_Tunnel:Heat_Ex_Div_Valve:Dem Pos" -> [w1068]
          tunnel: w1045 -> [w1063]
          tunnel: [w1061] -> w1043
          stop <- TRUE stop-if-true
          n432 = Not Equal?(x=w1066, y=w1067) -> (x != y?=w1064:bool)
          n433 = Compound Arithmetic op=OR(w1064, invert w1063) -> (w1062:bool)
          n434 = Build Array(w1068) -> (w1069:string[])
          n435 = Build Array(w1066) -> (w1070:dbl[])
          n436 = case shown="True" w1062 {
            tunnel: w1070 -> [_ w1074]
            tunnel: w1069 -> [_ w1073]
            tunnel: [string[] [] ("Scan Comments") w1072] -> w1061
            frame False {
            }
            frame True {
              n437 = call "ASYNC_Adam_server.vi"("Values"=w1074, "Channel Names"=w1073) -> ("Scan Comments"=w1072:string[])  [unwired: 1 in, 2 out]
            }
          }
        }
        n438 = Concatenate Strings(w1043) -> (w1041:string)
      }
      frame #30 {
        n439 = call "Read_value_of_earlier_Ch.vi"("Desired Ch to Read"="EnFlo_Tunnel:Safety_Loop:Status", "Ch names"=w1077, "Present scan array"=w1078) -> ("Value"=w1081:dbl, "Scan comment"=w1076:string)  [unwired: 1 in]
        n440 = Less?(x=w1081, y=0.5) -> (x < y?=w1075:bool)
        n441 = And(x=w1082, y=w1075) -> (x .and. y?=w1085:bool)
        n442 = case shown="True" w1085 {
          tunnel: ["" w1091] -> w1084
          frame False {
          }
          frame True {
            w1088 = string[] ["EnFlo_Tunnel:Bus Bar + Heaters:Enable", "EnFlo_Tunnel:Heater:Enable"] ("appended array")
            n443 = Array Size(array=w1088) -> (size(s)=w1089:i32)
            n444 = Initialize Array(0.0, w1089) -> (w1087:dbl[])
            n445 = call "ASYNC_Adam_server.vi"("Values"=w1087, "Channel Names"=w1088) -> ("Scan Comments"=w1092:string[])  [unwired: 1 in, 2 out]
            n446 = Index Array(array=w1092, index=0) -> (element=w1091:string)
          }
        }
        n447 = Concatenate Strings(w1084, w1076) -> (w1083:string)
      }
      frame #31 {
        w1095 = "EnFlo_Tunnel:Power:Chiller_Pump_Floor" ("Ch Name")
        n448 = case shown="True" w1096 {
          tunnel: w1101 -> [_ w1111]
          tunnel: w1100 -> [_ w1110]
          tunnel: [FALSE w1108] -> w1099
          tunnel: ["" w1104] -> w1097
          tunnel: w1095 -> [_ w1107]
          frame False {
          }
          frame True {
            n449 = call "Read_value_of_earlier_Ch.vi"("Desired Ch to Read"=w1107, "Ch names"=w1110, "Present scan array"=w1111) -> ("Value"=w1116:dbl, "Scan comment"=w1106:string)  [unwired: 1 in]
            n450 = call "Read_value_of_earlier_Ch.vi"("Desired Ch to Read"="EnFlo_Tunnel:Floor_Cooling:Enable", "Ch names"=w1110, "Present scan array"=w1111) -> ("Value"=w1113:dbl, "Scan comment"=w1105:string)  [unwired: 1 in]
            n451 = Concatenate Strings(w1106, w1105) -> (w1104:string)
            n452 = Greater?(x=w1116, y=0.5) -> (0:w1109:bool)
            n453 = Less?(x=w1113, y=0.5) -> (x < y?=w1112:bool)
            n454 = And(x=w1109, y=w1112) -> (x .and. y?=w1108:bool)
          }
        }
        n455 = case shown="True" w1099 {
          tunnel: ["" w1120] -> w1098
          tunnel: w1095 -> [_ w1119]
          frame False {
          }
          frame True {
            n456 = Build Array(0.0) -> (w1124:dbl[])
            n457 = Build Array(w1119) -> (w1125:string[])
            n458 = call "ASYNC_Adam_server.vi"("Values"=w1124, "Channel Names"=w1125) -> ("Scan Comments"=w1121:string[])  [unwired: 1 in, 2 out]
            n459 = Index Array(array=w1121, index=0) -> (element=w1120:string)
          }
        }
        n460 = Concatenate Strings(w1097, w1098) -> (w1094:string)
      }
      frame #32 {
        w1159 = "EnFlo_Tunnel:Power:Chiller_Pump_Exchanger"
        n461 = Greater?(x=w1163, y=25.0) -> (0:w1134:bool)
        n462 = Greater?(x=w1168, y=0.5) -> (0:w1164:bool)
        n463 = Compound Arithmetic op=AND(invert w1126, w1127, w1128, w1164, w1160) -> (w1132:bool)
        n464 = feedback #6() -> (w1136:dbl[])  [unwired: 1 in]
        n465 = call "Read_value_of_earlier_Ch.vi"("Desired Ch to Read"=w1159, "Ch names"=w1149, "Present scan array"=w1150) -> ("Value"=w1158:dbl, "Scan comment"=w1156:string)  [unwired: 1 in]
        n466 = call "Read_Earlier_Channels.vi"("Present scan array"=w1150, "Ch names"=w1149, "Desired Channels"=string[] ["EnFlo_Tunnel:Chilled Water:Return", "EnFlo_Tunnel:Chilled Water:Supply", "EnFlo_Tunnel:Speed:Dem Velocity", "EnFlo_Tunnel:Reference:Velocity"]) -> ("Index 0"=w1147:dbl, "Index 1"=w1146:dbl, "Index 2"=w1142:dbl, "Index 3"=w1141:dbl)  [unwired: 2 out]
        n467 = Build Array(w1159) -> (w1153:string[])
        n468 = Subtract(x=w1147, y=w1146) -> (x-y=w1145:dbl)
        n469 = call "In_Range_check.vi"("±"=0.25, "%"=30.0, "Mode"=In_Range."% & ±", "Value"=w1141, "Setpoint"=w1142) -> ("In Range"=w1129:bool)  [unwired: 2 in]
        n470 = Compound Arithmetic op=AND(w1129, w1134) -> (w1133:bool)
        n471 = call "On_Off_with_hysteresis.vi"("Shift In"=w1136, "History length"=100, "New Value"=w1133) -> ("Shift Out"=w1137:dbl[], "Output State"=w1131:bool)  [unwired: 3 in]
        n472 = feedback-in #6(w1137) -> ()
        n473 = And(x=w1132, y=w1131) -> (x .and. y?=w1130:bool)
        n474 = Divide(x=w1145, y=5.0) -> (x/y=w1143:dbl)
        n475 = case shown="True" w1130 {
          tunnel: w1163 -> [_ w1191]
          tunnel: w1162 -> [_ w1194]
          tunnel: [0.0 w1192] -> w1161
          tunnel: w1143 -> [_ w1184]
          frame False {
          }
          frame True {
            w1181 = 0.0 ("lower limit")
            n476 = feedback #7() -> (w1186:dbl[])  [unwired: 1 in]
            n477 = call "Running_Ch_Average.vi"("Shift In"=w1186, "History length"=120, "Reset Average after Seconds"=120.0, "New Value"=w1191) -> ("Shift Out"=w1187:dbl[], "mean"=w1190:dbl)  [unwired: 1 in, 1 out]
            n478 = feedback-in #7(w1187) -> ()
            n479 = Greater?(x=w1194, y=3.0) -> (0:w1195:bool)
            n480 = case shown="False" w1195 {
              tunnel: w1190 -> [w1200 w1210]
              tunnel: [w1198 w1208] -> w1185
              frame False {
                w1199 = 50.0 ("y")
                n481 = Greater?(x=w1200, y=w1199) -> (0:w1197:bool)
                n482 = case shown="False" w1197 {
                  tunnel: w1200 -> [_ w1206]
                  tunnel: w1199 -> [_ w1205]
                  tunnel: [0.0 w1202] -> w1198
                  frame False {
                  }
                  frame True {
                    n483 = Subtract(x=w1206, y=w1205) -> (x-y=w1204:dbl)
                    n484 = Multiply(x=w1204, y=2.0) -> (x*y=w1202:dbl)
                  }
                }
              }
              frame True {
                w1209 = 75.0 ("y")
                n485 = Greater?(x=w1210, y=w1209) -> (0:w1207:bool)
                n486 = case shown="True" w1207 {
                  tunnel: w1210 -> [_ w1216]
                  tunnel: w1209 -> [_ w1215]
                  tunnel: [0.0 w1212] -> w1208
                  frame False {
                  }
                  frame True {
                    n487 = Subtract(x=w1216, y=w1215) -> (x-y=w1214:dbl)
                    n488 = Multiply(x=w1214, y=4.0) -> (x*y=w1212:dbl)
                  }
                }
              }
            }
            n489 = Multiply(x=w1184, y=w1185) -> (x*y=w1182:dbl)
            n490 = feedback #8() -> (w1179:dbl[])  [unwired: 1 in]
            n491 = Greater?(x=w1182, y=15.0) -> (0:w1177:bool)
            n492 = call "On_Off_with_hysteresis.vi"("Shift In"=w1179, "History length"=30, "New Value"=w1177) -> ("Shift Out"=w1178:dbl[], "Output State"=w1176:bool)  [unwired: 3 in]
            n493 = feedback-in #8(w1178) -> ()
            n494 = Select(t=w1182, s=w1176, f=w1181) -> (s? t:f=w1180:dbl)
            n495 = In Range and Coerce(upper limit=100.0, x=w1180, lower limit=w1181) -> (coerced(x)=w1192:dbl)  [unwired: 1 out]
          }
        }
        n496 = Not Equal?(x=w1161, y=w1158) -> (x != y?=w1152:bool)
        n497 = Compound Arithmetic op=OR(w1152, invert w1166) -> (w1151:bool)
        n498 = Build Array(w1161) -> (w1154:dbl[])
        n499 = case shown="True" w1151 {
          tunnel: w1154 -> [_ w1173]
          tunnel: w1153 -> [_ w1172]
          tunnel: ["" w1170] -> w1157
          frame False {
          }
          frame True {
            n500 = call "ASYNC_Adam_server.vi"("Values"=w1173, "Channel Names"=w1172) -> ("Scan Comments"=w1171:string[])  [unwired: 1 in, 2 out]
            n501 = Index Array(array=w1171) -> (element=w1170:string)  [unwired: 1 in]
          }
        }
        n502 = Concatenate Strings(w1157, w1156) -> (w1155:string)
      }
      frame #33 {
        # "To automatically control the request for the University Stall chiller to run."
        n503 = while {
          tunnel: w1221 -> [w1230]
          tunnel: w1220 -> [w1231]
          shift-right: [w1225] -> _
          shift-left: _ -> [w1240]
          shift-left: _ -> [w1239]
          shift-left: _ -> [w1238]
          tunnel: [w1229] -> w1219
          tunnel: [w1228] -> w1218
          stop <- FALSE continue-if-true
          n504 = Build Array("Aero_Tunnel:Motor:Enable" ("Desired Ch to Read"), "EnFlo_Tunnel:Chiller_Pump:Running" ("Desired Ch to Read")) -> (w1232:string[])
          n505 = call "Read_Earlier_Channels.vi"("Present scan array"=w1230, "Ch names"=w1231, "Desired Channels"=w1232) -> ("Scan comments"=w1228:string, "Index 0"=w1227:dbl, "Index 1"=w1224:dbl)  [unwired: 3 out]
          n506 = Greater?(x=w1227, y=0.5) -> (0:w1223:bool)
          n507 = Greater?(x=w1224, y=0.5) -> (0:w1222:bool)
          n508 = Or(x=w1223, y=w1222) -> (x .or. y?=w1225:bool)
          n509 = Compound Arithmetic op=AND(w1225, w1240, invert w1239, invert w1238) -> (w1236:bool)
          n510 = Compound Arithmetic op=AND(invert w1225, invert w1240, w1239, w1238) -> (w1237:bool)
          n511 = Or(x=w1236, y=w1237) -> (x .or. y?=w1235:bool)
          n512 = case shown="True" w1235 {
            tunnel: w1225 -> [_ w1249]
            tunnel: [string[] [] ("Scan Comments") w1244] -> w1229
            frame False {
            }
            frame True {
              n513 = case shown="False" w1249 {
                tunnel: [string[] ["University:Chilled Water:Requested"] ("Channel Names") string[] ["University:Chilled Water:Requested"] ("Channel Names")] -> w1248
                tunnel: [1.0 ("y") 0.0 ("y")] -> w1245
                frame True {
                }
                frame False {
                }
              }
              n514 = Array Size(array=w1248) -> (size(s)=w1246:i32)
              n515 = Initialize Array(w1245, w1246) -> (w1247:dbl[])
              n516 = call "ASYNC_Adam_server.vi"("Values"=w1247, "Channel Names"=w1248) -> ("Scan Comments"=w1244:string[])  [unwired: 1 in, 2 out]
            }
          }
        }
        n517 = Concatenate Strings(w1219, w1218) -> (w1217:string)
      }
      frame #34 {
        # "Exercise the floor cooling valve once a week"
        n518 = while {
          shift-right: [w1258] -> _
          shift-left: _ -> [w1263]
          tunnel: w1256 -> [w1258]
          tunnel: w1255 -> [w1260]
          tunnel: [w1257] -> w1254
          stop <- TRUE stop-if-true
          n519 = Not Equal?(x=w1258, y=w1263) -> (x != y?=w1261:bool)
          n520 = Compound Arithmetic op=AND(w1261, w1260) -> (w1259:bool)
          n521 = case shown="True" w1259 {
            tunnel: w1258 -> [_ w1270]
            tunnel: ["" w1265] -> w1257
            frame False {
            }
            frame True {
              n522 = Select(t=1.0, s=w1270, f=0.0) -> (s? t:f=w1271:dbl)
              n523 = Build Array(w1271) -> (w1274:dbl[])
              n524 = Build Array("EnFlo_Tunnel:Floor_Cooling:Enable") -> (w1273:string[])
              n525 = call "ASYNC_Adam_server.vi"("Values"=w1274, "Channel Names"=w1273) -> ("Scan Comments"=w1266:string[])  [unwired: 1 in, 2 out]
              n526 = Index Array(array=w1266, index=0) -> (element=w1265:string)
            }
          }
        }
      }
      frame #35 {
        n527 = Build Array("GMU:CO2_Low:Siren") -> (w1279:string[])
        n528 = Quotient & Remainder(x=w1292, y=15) -> (x-y*floor(x/y)=w1290:i32)  [unwired: 1 out]
        n529 = call "Get_Current_Scan_server.vi"("Desired Channels"=w1279) -> ("Ch Description Array"=w1296:T9[], "Numerical Values"=w1286:dbl[])  [unwired: 1 out]
        n530 = Equal To 0?(x=w1290) -> (x = 0?=w1289:bool)
        n531 = Select(t=1.0, s=w1289, f=0.0) -> (s? t:f=w1288:dbl)
        n532 = Index Array(array=w1296, index=0) -> (element=w1295:T9)
        n533 = Index Array(array=w1286, index=0) -> (element=w1275:dbl)
        n534 = Unbundle By Name(w1295) -> ("A"=w1294:dbl)
        n535 = Greater?(x=w1275, y=0.5) -> (0:w1282:bool)
        n536 = Greater?(x=w1294, y=0.5) -> (0:w1283:bool)
        n537 = Not Equal?(x=w1288, y=w1275) -> (x != y?=w1277:bool)
        n538 = Or(x=w1283, y=w1282) -> (x .or. y?=w1281:bool)
        n539 = Build Array(w1288) -> (w1278:dbl[])
        n540 = Compound Arithmetic op=AND(w1277, w1281) -> (w1276:bool)
        n541 = case shown="True" w1276 {
          tunnel: w1278 -> [_ w1305]
          tunnel: w1279 -> [_ w1304]
          tunnel: ["" w1301] -> w1280
          frame False {
          }
          frame True {
            n542 = call "ASYNC_Adam_server.vi"("Values"=w1305, "Channel Names"=w1304) -> ("Scan Comments"=w1302:string[])  [unwired: 1 in, 2 out]
            n543 = Index Array(array=w1302, index=0) -> (element=w1301:string)
          }
        }
      }
      frame #36 {
        n544 = global read "ADAM_Global.vi" "Channel States to Control"() -> (w1307:string[][])
        n545 = Index Array(array=w1307, index (col)=0 ("disabled index (col)")) -> (element=w1309:string[])  [unwired: 1 in]
        n546 = Index Array(array=w1307, index (col)=1 ("disabled index (col)")) -> (element=w1306:string[])  [unwired: 1 in]
        n547 = while {
          tunnel: w1315 -> [w1324]
          tunnel: w1314 -> [w1323]
          shift-right: [w1322] -> _
          shift-left: _ -> [w1321]
          tunnel: w1313 -> [w1320]
          tunnel: w1309 -> [w1319]
          tunnel: w1306 -> [w1318]
          tunnel: [w1316] -> w1312
          stop <- TRUE stop-if-true
          n548 = for {
            tunnel: w1324 -> [w1336]
            tunnel: w1323 -> [w1335]
            tunnel: [w1345] -> w1322 mode=indexing
            tunnel: w1321 -> [w1344]
            tunnel: w1320 -> [w1341]
            tunnel: w1319 -> [w1339] mode=indexing
            tunnel: w1318 -> [w1328] mode=indexing
            tunnel: [w1338] -> w1316 mode=indexing
            i -> [w1343]
            w1340 = 5000.0  # Off delay period (s)
            n549 = call "Read_value_of_earlier_Ch.vi"("Desired Ch to Read"=w1339, "Ch names"=w1335, "Present scan array"=w1336) -> ("Value"=w1348:dbl, "Scan comment"=w1338:string)  [unwired: 1 in]
            n550 = String Length(string=w1328) -> (length=w1326:i32)
            n551 = Greater?(x=w1348, y=0.5) -> (0:w1330:bool)
            n552 = Decrement(x=w1326) -> (x-1=w1327:i32)
            n553 = String Subset(string=w1328, length (rest)=w1327) -> (substring=w1325:string)  [unwired: 1 in]
            n554 = Concatenate Strings("Status:of:", w1325) -> (w1334:string)
            n555 = call "Read_value_of_earlier_Ch.vi"("Desired Ch to Read"=w1334, "Ch names"=w1335, "Present scan array"=w1336) -> ("Value"=w1329:dbl, "Scan comment"=w1333:string)  [unwired: 1 in]
            n556 = Empty String/Path?(string/path=w1333) -> (empty?=w1332:bool)
            n557 = case shown="True" w1332 {
              tunnel: [w1349 w1352] -> w1331
              tunnel: w1330 -> [w1349 w1351]
              tunnel: w1329 -> [_ w1354]
              frame False {
              }
              frame True {
                n558 = Less?(x=w1354, y=7.0) -> (x < y?=w1350:bool)
                n559 = Or(x=w1350, y=w1351) -> (x .or. y?=w1352:bool)
              }
            }
            n560 = Index Array(array=w1344, index=w1343) -> (element=w1342:cluster{"Time ":dbl, "Channel State":bool})
            n561 = call "Active Channels controller.vi"("Off delay period (s)"=w1340, "Current time"=w1341, "Shift In"=w1342, "Channels commencing with these characters"=w1328, "Control Channel State"=w1331, "Control on"=Channel_State_Control."Channel Name Starts with") -> ("Shift Out"=w1345:cluster{"Time ":dbl, "Channel State":bool})  [unwired: 5 in]
          }
        }
        n562 = Concatenate Strings(w1312) -> (w1311:string)
      }
      frame #37 {
        w1370 = "EnFlo_Tunnel:Temp:"
        n563 = global read "ADAM_Global.vi" "Active Ch names"() -> (w1371:string[])
        n564 = String Length(string=w1370) -> (length=w1372:i32)
        n565 = for {
          tunnel: w1371 -> [w1376] mode=indexing
          tunnel: w1372 -> [w1380]
          tunnel: w1370 -> [w1378]
          tunnel: w1369 -> [w1377]
          tunnel: w1368 -> [w1375]
          tunnel: [w1374] -> w1367 mode=indexing if=w1373
          n566 = String Subset(string=w1376, length (rest)=w1380) -> (substring=w1379:string)  [unwired: 1 out]
          n567 = Equal?(x=w1379, y=w1378) -> (x = y?=w1373:bool)
          n568 = case shown="True" w1373 {
            tunnel: w1377 -> [_ w1389]
            tunnel: w1376 -> [_ w1388]
            tunnel: w1375 -> [_ w1386]
            tunnel: [0.0 ("Output") w1383] -> w1374
            frame False {
            }
            frame True {
              n569 = Search 1D Array(1D array=w1389, element=w1388) -> (index of element=w1387:i32)  [unwired: 1 in]
              n570 = Index Array(array=w1386, index=w1387) -> (element=w1384:dbl)
              n571 = Not A Number/Path/Refnum?(number/path/refnum=w1384) -> (NaN/Path/Refnum?=w1385:bool)
              n572 = Select(t=0.0, s=w1385, f=w1384) -> (s? t:f=w1383:dbl)
            }
          }
        }
        n573 = Build Array("EnFlo_Tunnel:Max:Temp" ("Channel Name"), "EnFlo_Tunnel:Hot:Relay") -> (w1360:string[])
        n574 = Array Max & Min(array=w1367) -> (max value=w1364:dbl)  [unwired: 3 out]
        n575 = Greater?(x=w1364, y=38.0) -> (0:w1362:bool)
        n576 = Select(t=1.0, s=w1362, f=0.0) -> (s? t:f=w1355:dbl)
        n577 = Build Array(w1364, w1355) -> (w1361:dbl[])
        n578 = call "ASYNC_Adam_server.vi"("Values"=w1361, "Channel Names"=w1360) -> ("Scan Comments"=w1359:string[])  [unwired: 1 in, 2 out]
        n579 = Concatenate Strings(w1359) -> (w1358:string)
      }
      frame #38 {
        n580 = while {
          shift-right: [w1409] -> _
          shift-left: _ -> [w1410]
          tunnel: w1395 -> [w1408]
          tunnel: w1394 -> [w1407]
          tunnel: [w1406] -> w1391
          shift-right: [w1405] -> _
          shift-left: _ -> [w1402]
          tunnel: w1393 -> [w1404]
          tunnel: w1392 -> [w1403]
          shift-right: [w1401] -> _
          shift-left: _ -> [w1400]
          shift-right: [w1398] -> _
          shift-left: _ -> [w1397]
          tunnel: w1390 -> [w1396]
          stop <- TRUE stop-if-true
          # "Dem Pos"
          # "Meas Pos"
          # "Pre Dem Pos"
          # "approx Pos"
          # "Current"
          # "Dem"
          # "Run PID"
          n581 = stacked-sequence {
            seq-local: [w1424 _ _ _ _] -> [_ _ w1468 _ w1555]
            seq-local: [_ w1449 _ _ _] -> [_ _ w1465 _ _]
            seq-local: [_ w1448 _ _ _] -> [_ _ w1464 _ _]
            seq-local: [_ w1447 _ _ _] -> [_ _ w1463 _ _]
            seq-local: [w1414 _ _ _ _] -> [_ _ w1461 _ _]
            seq-local: [_ _ w1460 _ _] -> [_ _ _ w1539 w1554]
            seq-local: [_ w1438 _ _ _] -> [_ _ _ w1538 _]
            seq-local: [w1412 _ _ _ _] -> [_ _ w1458 w1533 _]
            seq-local: [_ _ _ w1536 _] -> [_ _ _ _ w1549]
            seq-local: [_ w1436 _ _ _] -> [_ _ _ w1534 _]
            seq-local: [_ _ w1457 _ _] -> [_ _ _ w1535 _]
            seq-local: [_ _ _ w1532 _] -> [_ _ _ _ w1548]
            tunnel: w1410 -> [w1423 _ _ _ _]
            tunnel: [w1422 _ _ _ _] -> w1409
            tunnel: w1408 -> [w1417 w1454 w1467 _ w1553]
            tunnel: w1407 -> [w1416 w1453 w1466 _ w1552]
            tunnel: [_ _ w1462 _ _] -> w1406
            tunnel: [_ _ _ _ w1556] -> w1405
            tunnel: w1402 -> [w1413 _ _ _ w1559]
            tunnel: w1404 -> [w1421 _ w1456 _ _]
            tunnel: w1403 -> [_ _ w1459 _ _]
            tunnel: [_ w1444 _ _ _] -> w1401
            tunnel: w1400 -> [_ w1443 _ _ _]
            tunnel: "EnFlo_Tunnel:Chilled Water:Valve Dem Pos" -> [w1415 _ _ _ w1550]
            tunnel: [_ _ _ w1541 _] -> w1398
            tunnel: w1397 -> [_ _ _ w1540 _]
            tunnel: w1396 -> [_ _ w1455 _ _]
            frame #0 {
              n582 = Array Size(array=w1413) -> (size(s)=w1419:i32)
              n583 = Greater Than 0?(x=w1419) -> (x > 0?=w1418:bool)
              n584 = Subtract(x=w1421, y=w1423) -> (x-y=w1427:dbl)
              n585 = case shown="True" w1418 {
                tunnel: w1417 -> [w1431 _]
                tunnel: w1416 -> [w1430 _]
                tunnel: w1415 -> [w1429 _]
                tunnel: [w1428 w1432] -> w1414
                tunnel: w1413 -> [_ w1433]
                tunnel: [w1428 w1434] -> w1412
                frame False {
                  n586 = call "Read_value_of_earlier_Ch.vi"("Desired Ch to Read"=w1429, "Ch names"=w1430, "Present scan array"=w1431) -> ("Value"=w1428:dbl)  [unwired: 1 in, 1 out]
                }
                frame True {
                  n587 = Index Array(array=w1433) -> (element=w1434:dbl)  [unwired: 1 in]
                  n588 = call "Mean_fr_NaN_data.vi"("Data"=w1433) -> ("Mean value"=w1432:dbl)  [unwired: 1 out]
                }
              }
              n589 = Greater?(x=w1427, y=10.0) -> (0:w1426:bool)
              n590 = Not A Number/Path/Refnum?(number/path/refnum=w1427) -> (NaN/Path/Refnum?=w1425:bool)
              n591 = Or(x=w1425, y=w1426) -> (x .or. y?=w1424:bool)
              n592 = Select(t=w1421, s=w1424, f=w1423) -> (s? t:f=w1422:dbl)
            }
            frame #1 {
              n593 = Build Array("EnFlo_Tunnel:Chilled Water:Dem Temp", "EnFlo_Tunnel:Chilled Water:Supply", "EnFlo_Tunnel:Chilled Water:Valve Meas Pos") -> (w1450:string[])
              n594 = call "Read_Earlier_Channels.vi"("Present scan array"=w1454, "Ch names"=w1453, "Desired Channels"=w1450) -> ("Scan comments"=w1447:string, "Index 0"=w1449:dbl, "Index 1"=w1448:dbl, "Index 2"=w1435:dbl)  [unwired: 2 out]
              n595 = Build Array (concatenate)(w1435, w1443) -> (w1437:dbl[])
              n596 = Array Max & Min(array=w1437) -> (max value=w1442:dbl, min value=w1441:dbl)  [unwired: 2 out]
              n597 = Subtract(x=w1442, y=w1441) -> (x-y=w1440:dbl)
              n598 = Less?(x=w1440, y=0.06) -> (x < y?=w1438:bool)
              n599 = call "Mean_fr_NaN_data.vi"("Data"=w1437) -> ("Mean value"=w1436:dbl)  [unwired: 1 out]
              n600 = Array Subset(array=w1437, length=7 ("History Length")) -> (w1444:dbl[])  [unwired: 1 in]
            }
            frame #2 {
              n601 = case shown="True" w1468 {
                tunnel: w1467 -> [_ w1491]
                tunnel: w1466 -> [_ w1490]
                tunnel: w1465 -> [_ w1488]
                tunnel: w1458 -> [w1471 w1487]
                tunnel: [w1471 w1486] -> w1460
                tunnel: w1464 -> [_ w1485]
                tunnel: w1463 -> [w1470 w1484]
                tunnel: [w1470 w1482] -> w1462
                tunnel: w1461 -> [_ w1479]
                tunnel: w1459 -> [_ w1478]
                tunnel: [FALSE w1476] -> w1457
                tunnel: w1456 -> [_ w1473]
                tunnel: w1455 -> [_ w1472]
                frame False {
                }
                frame True {
                  n602 = call "Read_Earlier_Channels.vi"("Present scan array"=w1491, "Ch names"=w1490, "Desired Channels"=string[] ["EnFlo_Tunnel:Chiller_Pump:Running", "Uni:Chilled Water:Temp", "EnFlo_Tunnel:Chiller_Pump:Enable", "EnFlo_Tunnel:Chilled Water:Return"] ("appended array")) -> ("Scan comments"=w1483:string, "Index 0"=w1480:dbl, "Index 1"=w1477:dbl, "Index 2"=w1475:dbl, "Index 3"=w1474:dbl)  [unwired: 1 out]
                  n603 = Greater?(x=w1480, y=0.5) -> (0:w1476:bool)
                  n604 = case shown="True" w1476 {
                    tunnel: [w1495 w1516] -> w1486
                    tunnel: w1488 -> [_ w1514]
                    tunnel: w1485 -> [_ w1517]
                    tunnel: w1487 -> [_ w1513]
                    tunnel: w1477 -> [_ w1515]
                    tunnel: w1479 -> [_ w1512]
                    tunnel: w1478 -> [_ w1511]
                    tunnel: w1472 -> [_ w1510]
                    tunnel: w1475 -> [w1494 _]
                    tunnel: w1474 -> [_ w1509]
                    tunnel: w1473 -> [_ w1508]
                    frame False {
                      n605 = Greater?(x=w1494, y=0.5) -> (0:w1492:bool)
                      n606 = case shown="True" w1492 {
                        tunnel: [w1506 0.0 ("f")] -> w1495
                        frame False {
                          n607 = Seconds To Date/Time() -> (date time rec=w1496:T8)  [unwired: 2 out]
                          n608 = Unbundle By Name(w1496) -> ("day of week"=w1501:i32, "hour"=w1503:i32)
                          n609 = Less?(x=w1503, y=3) -> (x < y?=w1498:bool)
                          n610 = Equal?(x=7, y=w1501) -> (x = y?=w1499:bool)
                          n611 = And(x=w1499, y=w1498) -> (x .and. y?=w1497:bool)
                          n612 = Select(t=0.0, s=w1497, f=100.0) -> (s? t:f=w1506:dbl)
                        }
                        frame True {
                        }
                      }
                    }
                    frame True {
                      n613 = case shown="False" w1511 {
                        tunnel: w1517 -> [_ w1531]
                        tunnel: [w1518 w1528] -> w1516
                        tunnel: w1515 -> [_ w1525]
                        tunnel: w1514 -> [_ w1529]
                        tunnel: w1513 -> [_ w1530]
                        tunnel: w1512 -> [_ _]
                        tunnel: w1510 -> [w1521 w1526]
                        tunnel: w1509 -> [_ w1523]
                        tunnel: w1508 -> [_ w1522]
                        frame False {
                          n614 = Select(t=100.0 ("Max"), s=w1521, f=0.0) -> (s? t:f=w1518:dbl)
                        }
                        frame True {
                          w1527 = 100.0  # Max
                          n615 = call "Chilled water mixing valve PID.vi"("Setpoint"=w1529, "EnFlo_Tunnel:Chilled Water:Return"=w1523, "Previous Scan Value"=w1530, "Present Value"=w1531, "Uni Chilled Water Temperature"=w1525, "Current Time"=w1522) -> ("Dem Output"=w1524:dbl)
                          n616 = Select(t=w1527, s=w1526, f=w1524) -> (s? t:f=w1528:dbl)
                        }
                      }
                    }
                  }
                  n617 = Concatenate Strings(w1483, w1484) -> (w1482:string)
                }
              }
            }
            frame #3 {
              n618 = Select(t=w1534, s=w1535, f=w1533) -> (s? t:f=w1532:dbl)
              n619 = Build Array (concatenate)(w1539, w1540) -> (w1542:dbl[])
              n620 = Array Max & Min(array=w1542) -> (max value=w1546:dbl, min value=w1545:dbl)  [unwired: 2 out]
              n621 = Subtract(x=w1546, y=w1545) -> (x-y=w1544:dbl)
              n622 = Less?(x=w1544, y=0.1) -> (x < y?=w1537:bool)
              n623 = And(x=w1538, y=w1537) -> (x .and. y?=w1536:bool)
              n624 = Array Subset(array=w1542, length=10 ("History Length")) -> (w1541:dbl[])  [unwired: 1 in]
            }
            frame #4 {
              n625 = Build Array (concatenate)(w1554, w1559) -> (w1557:dbl[])
              n626 = Build Array(w1550) -> (w1551:string[])
              n627 = case shown="True" w1555 {
                tunnel: w1554 -> [_ w1560]
                tunnel: w1553 -> [_ _]
                tunnel: w1552 -> [_ _]
                tunnel: w1551 -> [_ w1568]
                tunnel: w1548 -> [_ w1566]
                tunnel: w1549 -> [_ w1565]
                frame False {
                }
                frame True {
                  w1561 = 3.0 ("upper limit")
                  n628 = Subtract(x=w1566, y=w1560) -> (x-y=w1567:dbl)
                  n629 = Absolute Value(x=w1567) -> (abs(x)=w1564:dbl)
                  n630 = In Range and Coerce(upper limit=w1561, x=w1564, lower limit="Valve Tolerance") -> (In Range?=w1562:bool)  [unwired: 1 out]
                  n631 = And(x=w1565, y=w1562) -> (x .and. y?=w1569:bool)
                  n632 = case shown="False" w1569 {
                    tunnel: w1564 -> [w1574 w1581]
                    tunnel: w1568 -> [w1570 w1580]
                    tunnel: w1567 -> [_ w1579]
                    tunnel: w1560 -> [w1571 w1578]
                    tunnel: w1561 -> [w1573 _]
                    frame False {
                      n633 = Greater?(x=w1574, y=w1573) -> (0:w1572:bool)
                      n634 = case shown="True" w1572 {
                        tunnel: w1571 -> [_ w1576]
                        tunnel: w1570 -> [_ w1575]
                        frame False {
                        }
                        frame True {
                          n635 = Build Array(w1576) -> (w1577:dbl[])
                          n636 = call "ASYNC_Adam_server.vi"("Values"=w1577, "Channel Names"=w1575) -> ()  [unwired: 1 in, 3 out]
                        }
                      }
                    }
                    frame True {
                      n637 = stacked-sequence {
                        tunnel: w1581 -> [_ w1596 _]
                        tunnel: w1580 -> [w1588 _ w1602]
                        tunnel: w1579 -> [w1587 _ _]
                        tunnel: w1578 -> [w1584 _ w1600]
                        frame #0 {
                          n638 = Greater Than 0?(x=w1587) -> (x > 0?=w1585:bool)
                          n639 = case shown="False" w1585 {
                            tunnel: w1584 -> [w1591 w1594]
                            tunnel: 2.5 ("x") -> [w1590 w1593]
                            tunnel: [w1589 w1592] -> w1583
                            frame False {
                              n640 = Add(x=w1590, y=w1591) -> (x+y=w1589:dbl)
                            }
                            frame True {
                              n641 = Subtract(x=w1594, y=w1593) -> (x-y=w1592:dbl)
                            }
                          }
                          n642 = Build Array(w1583) -> (w1582:dbl[])
                          n643 = call "ASYNC_Adam_server.vi"("Values"=w1582, "Channel Names"=w1588) -> ()  [unwired: 2 in, 2 out]
                        }
                        frame #1 {
                          n644 = Multiply(x=w1596, y=1500.0) -> (x*y=w1597:dbl)
                          n645 = Subtract(x=w1597, y=60.0) -> (x-y=w1599:dbl)
                          n646 = Wait (ms)(milliseconds to wait=w1599) -> ()  [unwired: 1 out]
                        }
                        frame #2 {
                          n647 = Build Array(w1600) -> (w1601:dbl[])
                          n648 = call "ASYNC_Adam_server.vi"("Values"=w1601, "Channel Names"=w1602) -> ()  [unwired: 2 in, 2 out]
                        }
                      }
                    }
                  }
                }
              }
              n649 = Array Subset(array=w1557, length=150 ("History Length")) -> (w1556:dbl[])  [unwired: 1 in]
            }
          }
        }
      }
      frame #39 {
        n650 = Concatenate Strings(w1610, w1611, w1612, w1614, w1616, w1617, w1618, "", w1619, w1607, w1620, w1621, w1622, w1613, w1608, w1623, w1629, w1630, w1615, w1631, w1609, w1632, w1633, w1605, w1606, w1639, w1638, w1637, w1636, w1635, w1634, w1627, w1626, w1625, w1624, w1604) -> (→"Scan comment":string)
      }
    }
  }
